vi "GageAdvMultiRec8bit_Core.vi"(5 "Encoder feedback ref":refnum<vi>, 8 "error in":errorcluster, 9 "SignalBuffer queue in":refnum<queue>, 10 "GenericDAQ CtrlQueue in":refnum<queue>) -> (0 "error out":errorcluster)   [LabVIEW 2014]
uses:
  <instrlib>/GenericDAQ/VI/GenericDAQ_Ctrl_Queue.ctl
  <instrlib>/GenericDAQ/VI/GenericDAQ_State.ctl
  <instrlib>/GenericDAQ/VI/GenericDAQ_Signal.ctl
  <instrlib>/GageLv_uic/VI/Gage_Configs.ctl
  <instrlib>/GageLv_uic/VI/Gage_PrivateStats.ctl
  <instrlib>/GageLv_uic/VI/Gage_DAQStatus.ctl
  EncoderReadout/VI/EncoderReadout_PrivateStats.ctl
  EncoderReadout/VI/Encoder_State.ctl
  <instrlib>/GageLv_uic/VI/SetSecondaryDataVIRef_Typedef.ctl
  <vilib>/Utility/error.llb/Error Cluster From Error Code.vi
  <vilib>/ErrorRing/Error Ring.xnode
  <instrlib>/GageLv_uic/GageLv.lvlib
  <userlib>/Utility/ErrorLog_lib.lvlib
  EncoderReadout/EncoderReadout(NI-DAQmx).lvlib
  <instrlib>/GenericDAQ/GenericDAQ.lvlib
panel:
  out "element":T1
  out "Segment Count (1)":u32
  out "GenericDAQ State":T2
  out "ctrl elements":T3[](array[typedef])
  out "DynamicBuffer_Bak":refnum<queue>
  in  "SetPosition":dbl[](array[numeric])=[0.0, 0.0]
  out "pos_raw_data":dbl[][](array[numeric])
  out "volt conv. time":u32
  out "transfer time":u32
  in  "StartAll":bool
  in  "Get_ConfigAll":bool
  out "LiveStat":T4
  in  "Gage_Config":T6={"Acquisition"={"Sample Rate"=4000000000.0, "Mode"=0, "Start (0)"=0.0, "Depth"=8192.0, "Segment Size"=8192.0, "Trigger Delay"=0.0, "Trigger Timeout"=10.0, "Trigger Holdoff"=0.0, "Clock mode"=enum."Internal", "Segment"=1}, "Channels"=[{"Coupling"=0, "Differential Input"=FALSE, "Direct-to-ADC"=FALSE, "Range"=2000, "Impedance"=50, "DC Offset"=0, "Filter"=0}], "Trigger"={"Slope"=0, "Level"=25, "Source"=0, "External Range"=2000, "External Coupling"=0, "External"=TRUE, "Disable"=FALSE, "External Impedance"=0}, "Mode(Gage)"=enum."Continuous"} {"Trigger"."External Impedance" items=["50 Ohm", "HiZ"]; "Trigger"."External Coupling" items=["DC", "AC"]; "Trigger"."External Range" min=2000 max=10000 step=8000; "Trigger"."Slope" items=["Rising", "Falling"]; "Trigger"."Level" min=-100 max=100; "Trigger"."Source" min=0 max=64 step=1; "Channels"."Impedance" min=50 max=1000000 step=999950; "Channels"."Coupling" items=["DC", "AC"]; "Acquisition"."Start (0)" min=-1000000.0 max=0.0 step=16.0; "Acquisition"."Segment Size" min=256.0 step=128.0; "Acquisition"."Trigger Delay" min=0.0 step=128.0; "Acquisition"."Trigger Timeout" format="%.0p"; "Acquisition"."Trigger Holdoff" min=0.0 step=128.0; "Acquisition"."Depth" min=256.0 step=128.0; "Acquisition"."Mode" items=["Single", "Dual", "Quad", "Octal"]; "Acquisition"."Sample Rate" format="%.0p"}
  out "Graph":sgl[](graph)
  in  "fConfig":bool
  in  "Reset":bool
  in  "CloseAll":bool
  in  "Close":bool
  in  "Enumerate":bool
  in  "Open":bool
  in  "Quit":bool
  in  "Start":bool
  in  "ConfigAll":bool
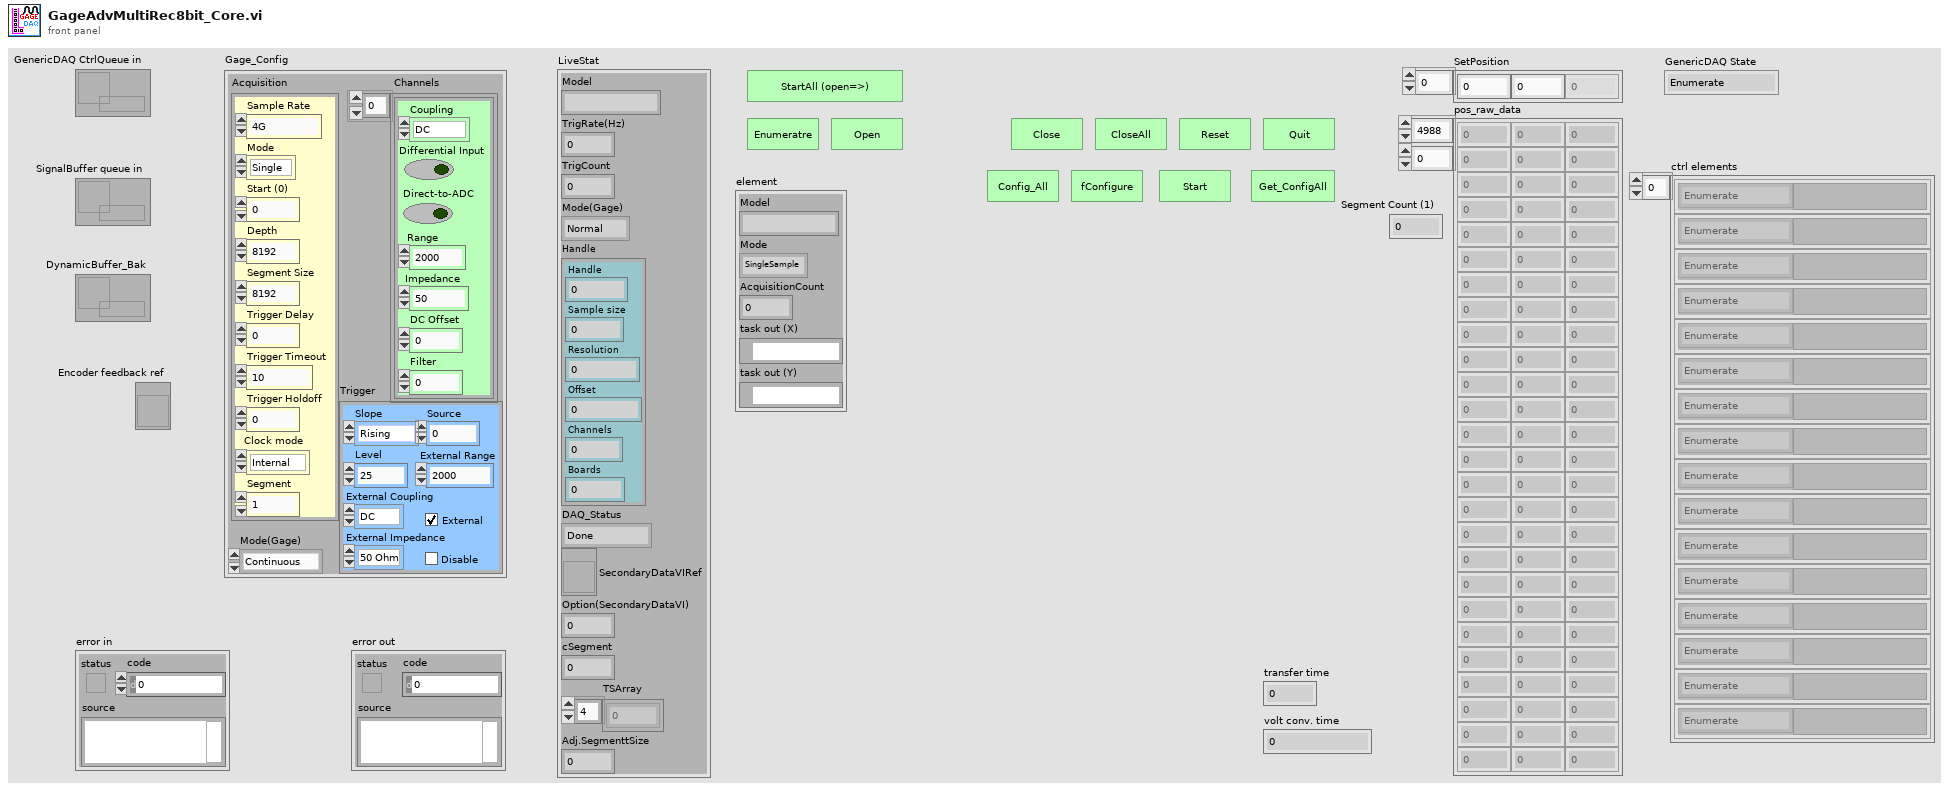
[diagram p1: front panel]
types:
  T1 = typedef "EncoderReadout(NI-DAQmx).lvlib/EncoderReadout_PrivateStats.ctl" = cluster{"Model":string, "Mode":enum16{"SingleSample", "NSamples", "Continuous"}, "AcquisitionCount":i32, "task out (X)":refnum<k21>, "task out (Y)":refnum<k21>}
  T2 = typedef "GenericDAQ.lvlib/GenericDAQ_State.ctl" = enum16{"Enumerate", "Open", "Close", "CloseAll", "Reset", "Quit", "==Settings==", "SetAcquisition_", "SetChannels_", "SetTrigger_", "SetAnalogTrigDetector_", "SetSegment#_", "SetAll_AcquChTrig_", "fConfigurate", "fStart", "GetStatus", "_WaitForDone/Idle", "_GetData", "GetAcquisition", "GetChannels", "GetTrigger", "GetAll_AcquChTrig", "Abort", "==Messaging==", "_PushDataOut", "GetStat_", "GetConfig_", "==ModeSetup==", "SetSignalBuffer_", "SetMode_", "SetSecondaryDataRef._", "SetDynamicBuffer_", "==AnalogOut==", "GetChannelCount_AO", "fStart_AO", "SetChEnable_AO", "SetConfig_AO", "SetFuncData_AO", "SetOffset_AO_", "SetMasterNode_AO", "SetStates_AO", "SetSymetry_AO", "SetTriggerSource_AO", "==Trigger==", "ManualTrigger", "===Sync===", "LineStart", "LineEnd", "FrameStart", "FrameEnd", "EOL_PassThrough", "SOL_PassThrough"}
  T3 = typedef "GenericDAQ.lvlib/GenericDAQ_Ctrl_Queue.ctl" = cluster{"GenericDAQ State":T2, "Variant":variant}
  T4 = typedef "GageLv.lvlib/Gage_PrivateStats.ctl" = cluster{"Model":string, "TrigRate(Hz)":dbl, "TrigCount":i32, "Mode(Gage)":enum16{"Normal", "Continuous", "MultiRecord", "HwAverage"}, "Handle":cluster{"Handle":u32, "Sample size":u32, "Resolution":i32, "Offset":i32, "Channels":u32, "Boards":u32}, "DAQ_Status":T5, "SecondaryDataVIRef":refnum<vi>, "Option(SecondaryDataVI)":i32, "cSegment":i32, "TSArray":dbl[], "Adj.SegmenttSize":dbl}
  T5 = typedef "GageLv.lvlib/Gage_DAQStatus.ctl" = enum16{"Done", "Armed", "Triggered", "Transfering"}
  T6 = typedef "GageLv.lvlib/Gage_Configs.ctl" = cluster{"Acquisition":cluster{"Sample Rate":dbl, "Mode":u16, "Start (0)":dbl, "Depth":dbl, "Segment Size":dbl, "Trigger Delay":dbl, "Trigger Timeout":dbl, "Trigger Holdoff":dbl, "Clock mode":enum16{"Internal", "External", "Reference"}, "Segment":u32}, "Channels":cluster{"Coupling":u16, "Differential Input":bool, "Direct-to-ADC":bool, "Range":u32, "Impedance":u32, "DC Offset":i32, "Filter":i32}[], "Trigger":cluster{"Slope":u16, "Level":i32, "Source":i32, "External Range":u32, "External Coupling":u16, "External":bool, "Disable":bool, "External Impedance":u16}, "Mode(Gage)":enum16{"Normal", "Continuous", "MultiRecord", "HwAverage"}}
  T7 = typedef "SetSecondaryDataVIRef_Typedef.ctl" = cluster{"SecondaryDataVIRef.":refnum<vi>, "Option":i32}
  T8 = cluster{"tickcount":u32, "Position":dbl[][], "Flag":enum16{"Normal", "MultiRecStart", "MultiRecEnd", "Reserved1", "Reserved2", "Reserved3"}}
  T9 = typedef "EncoderReadout(NI-DAQmx).lvlib/Encoder_State.ctl" = cluster{"EncoderReadout States":enum16{"Open", "Close", "Quit", "SetPosition", "SetPointsNum", "SetSyncChannel", "Start(Flush)", "GetPositions", "QueryStatus", "SetTimeout", "SetMode", "SetSignalOutputBuffer", "GetConfigs", "Wait", "Clear", "Stop", "FlushBuffer"}, "Variant":variant}
  T10 = typedef "GenericDAQ.lvlib/GenericDAQ_Signal.ctl" = cluster{"tickcount":u32, "Signal":sgl[], "SecondaryData":dbl[], "Flag":enum16{"Normal", "LineStart", "LineEnd", "FrameStart", "FrameEnd", "Reserved1", "Reserved2"}, "Segment#":i32}
  T11 = enum16{"Normal", "LineStart", "LineEnd", "FrameStart", "FrameEnd", "Reserved1", "Reserved2"}
  T12 = enum16{"Normal", "Continuous", "MultiRecord", "HwAverage"}
  T13 = cluster{"Handle":u32, "Sample size":u32, "Resolution":i32, "Offset":i32, "Channels":u32, "Boards":u32}
  T14 = cluster{"Sample Rate":dbl, "Mode":u16, "Start (0)":dbl, "Depth":dbl, "Segment Size":dbl, "Trigger Delay":dbl, "Trigger Timeout":dbl, "Trigger Holdoff":dbl, "Clock mode":enum16{"Internal", "External", "Reference"}, "Segment":u32}
  T15 = cluster{"Sample Rate":dbl, "Clock mode":enum16{"Internal", "External", "Reference"}, string, "Depth":dbl, "Segment Size":dbl, "Trigger Timeout":dbl, "Trigger Holdoff":dbl, "Trigger Delay":dbl}
  T16 = cluster{"Coupling":u16, "Differential Input":bool, "Direct-to-ADC":bool, "Range":u32, "Impedance":u32, "DC Offset":i32, "Filter":i32}[]
  T17 = cluster{string, "Differential Input":bool, "Direct-to-ADC":bool, "Range":u32, "Impedance":u32, "DC Offset":i32, "Filter":i32}
  T18 = cluster{"Slope":u16, "Level":i32, "Source":i32, "External Range":u32, "External Coupling":u16, "External":bool, "Disable":bool, "External Impedance":u16}
  T19 = cluster{string, "Level":i32, "Source":i32, "External Range":u32, string, "External":bool, "Disable":bool, string}
  T20 = cluster{string, "Level":i32, "Source":i32, "External Range":u32, string, "External":bool, "Disable":bool, string}[]
  T21 = cluster{"Handle":u32, "Sample Size":u32, "Resolution":i32, "Offset":i32, "Channels":u32, "Boards":u32}
  T22 = cluster{"Coupling":u16, "Differential Input":bool, "Direct-to-ADC":bool, "Range":u32, "Impedance":u32, "DC Offset":i32, "Filter":i32}
  T23 = cluster{"queue out":refnum<queue>, "queue out":refnum<queue>}
  T24 = typedef "Gage.lvlib/Gage_Configs.ctl" = cluster{"Acquisition":cluster{"Sample Rate":dbl, "Mode":u16, "Start (0)":dbl, "Depth":dbl, "Segment Size":dbl, "Trigger Delay":dbl, "Trigger Timeout":dbl, "Trigger Holdoff":dbl, "Clock mode":enum16{"Internal", "External", "Reference"}, "Segment":u32}, "Channels":cluster{"Coupling":u16, "Differential Input":bool, "Direct-to-ADC":bool, "Range":u32, "Impedance":u32, "DC Offset":i32, "Filter":i32}[], "Trigger":cluster{"Slope":u16, "Level":i32, "Source":i32, "External Range":u32, "External Coupling":u16, "External":bool, "Disable":bool, "External Impedance":u16}, "Mode(Gage)":enum16{"Normal", "Continuous", "MultiRecord", "HwAverage"}}
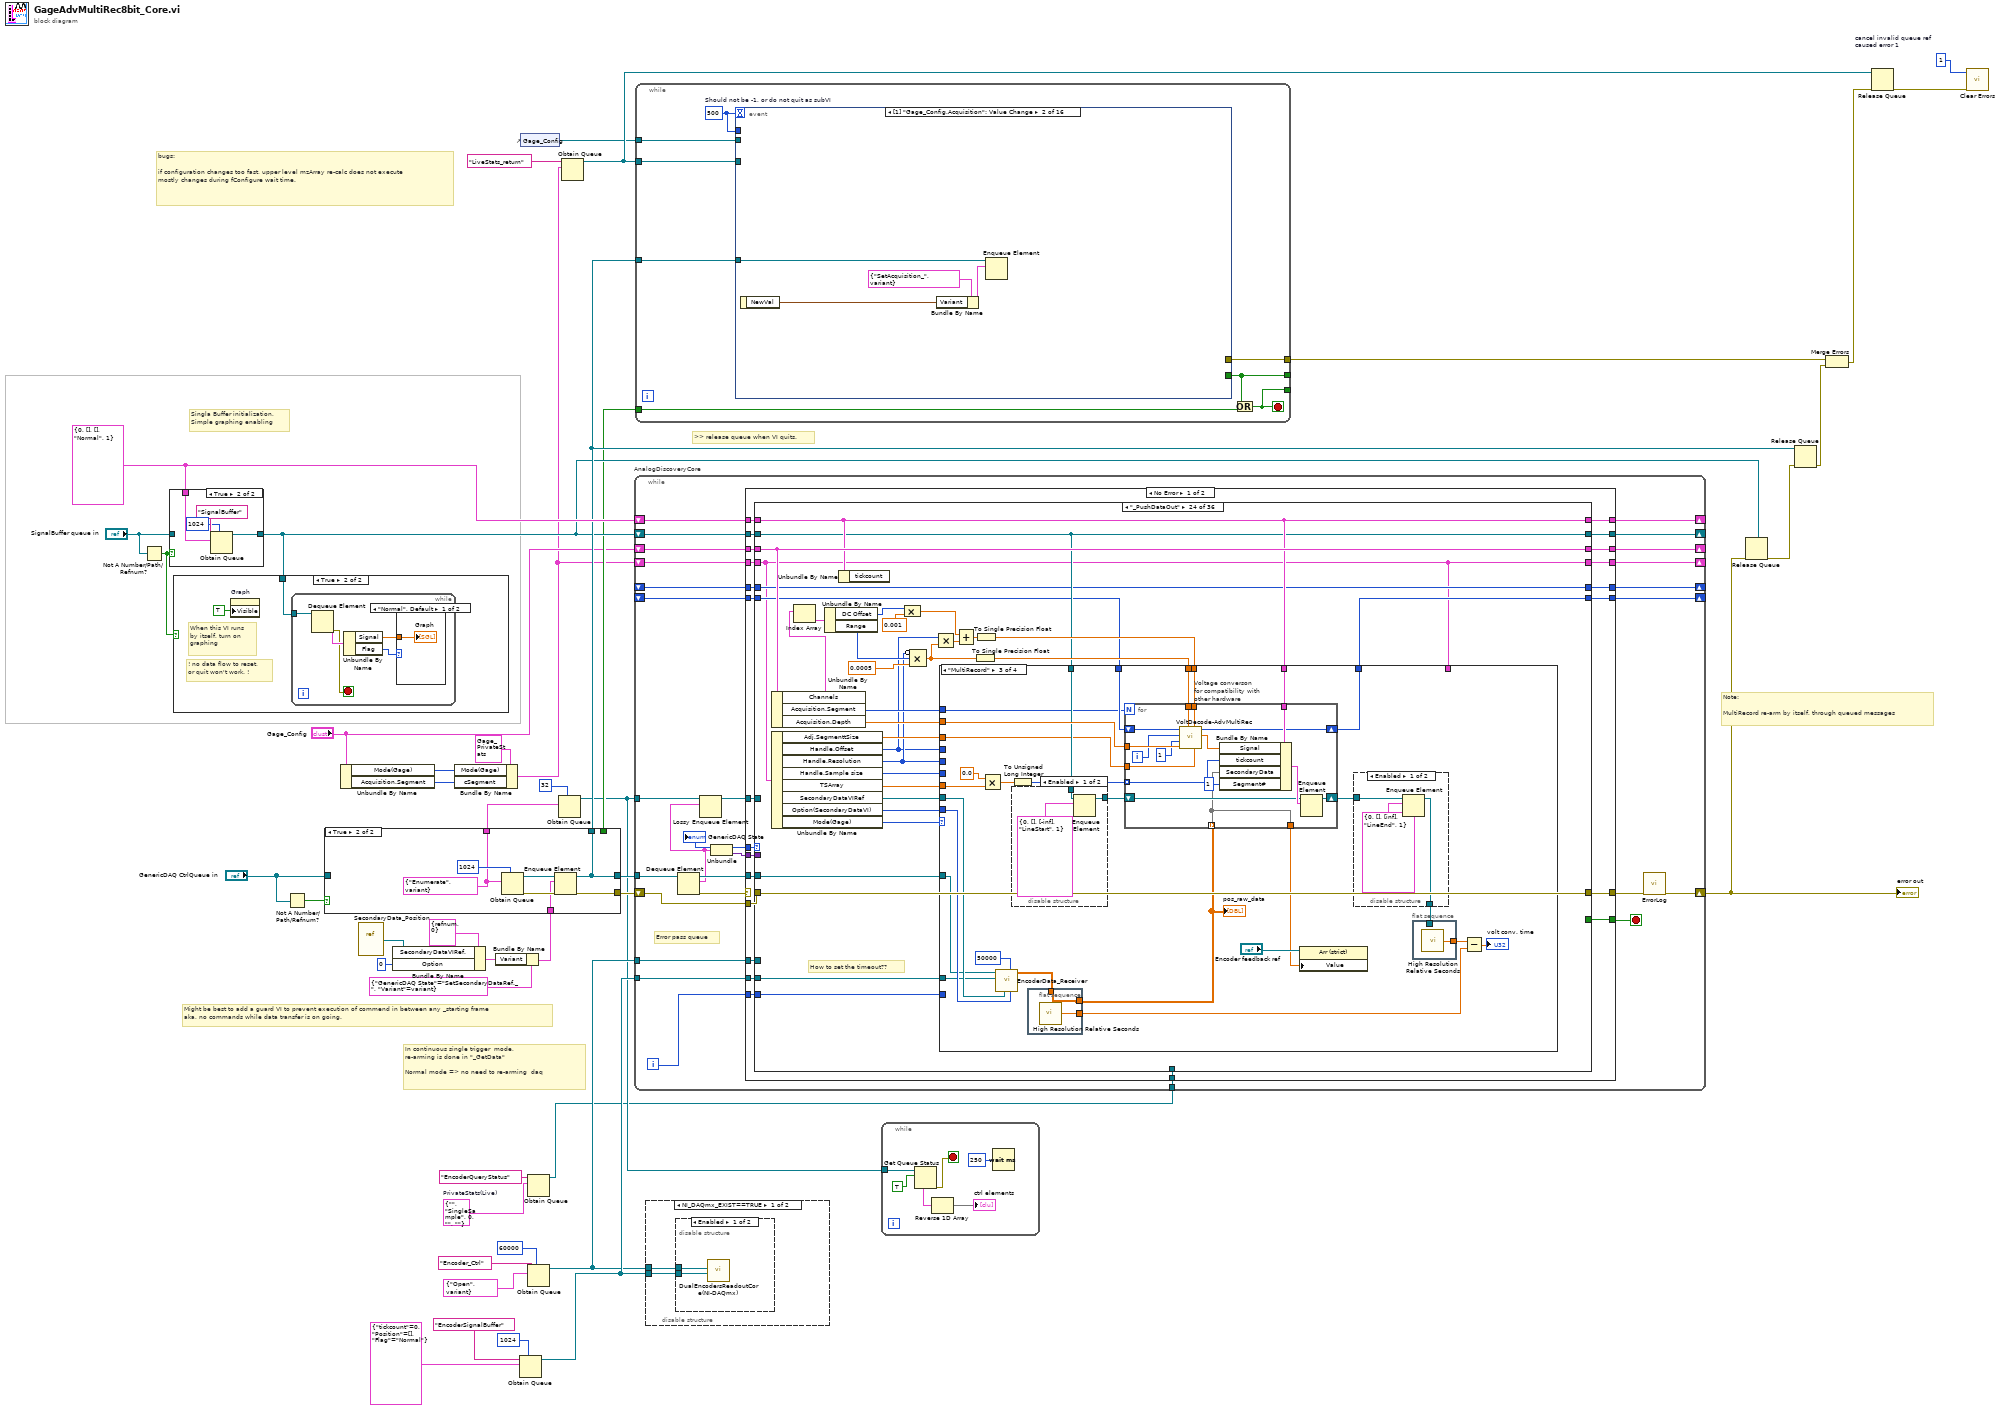
[diagram p0: block diagram]
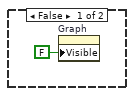
[diagram p4: hidden frame]
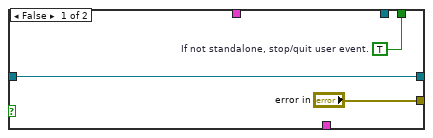
[diagram p7: hidden frame]
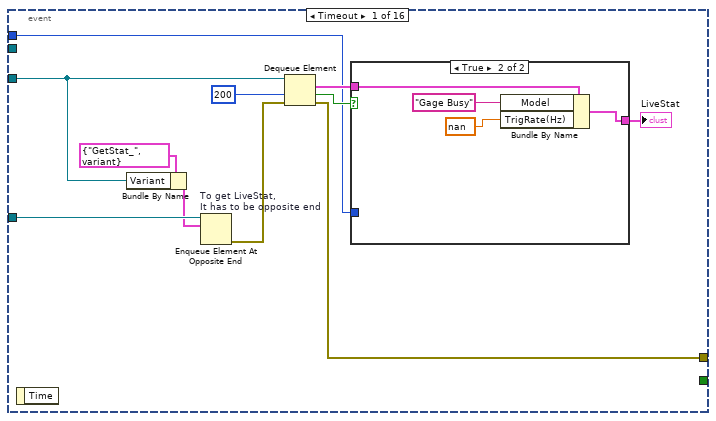
[diagram p8: hidden frame]
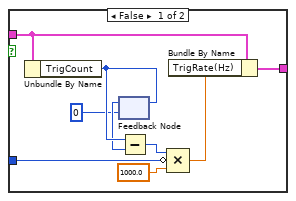
[diagram p9: hidden frame]
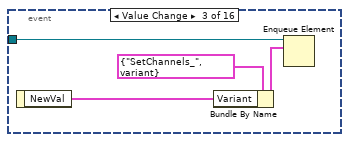
[diagram p10: hidden frame]
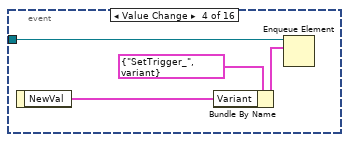
[diagram p11: hidden frame]
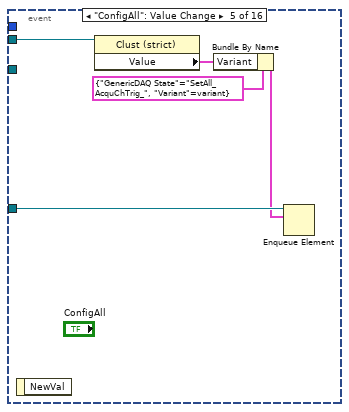
[diagram p12: hidden frame]
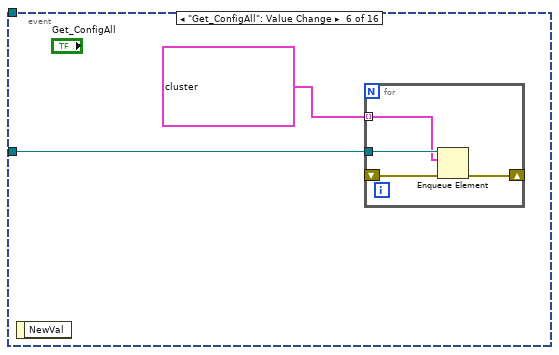
[diagram p13: hidden frame]
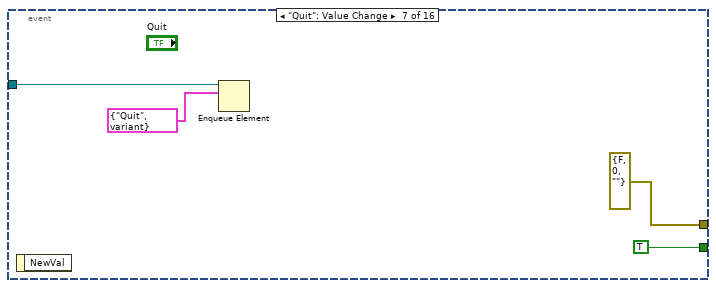
[diagram p14: hidden frame]
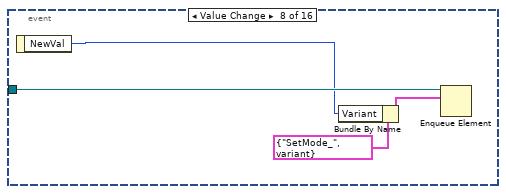
[diagram p15: hidden frame]
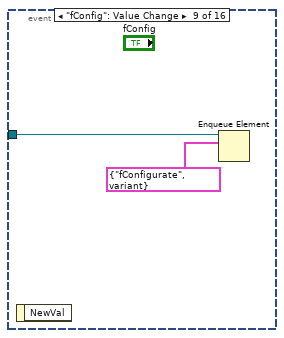
[diagram p16: hidden frame]
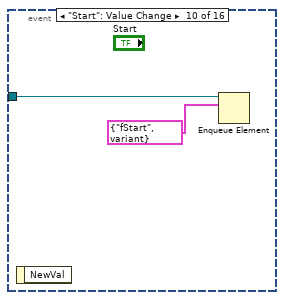
[diagram p17: hidden frame]
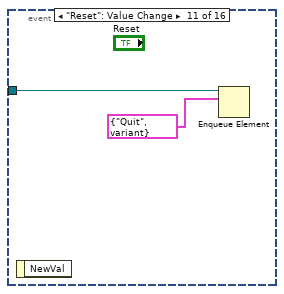
[diagram p18: hidden frame]
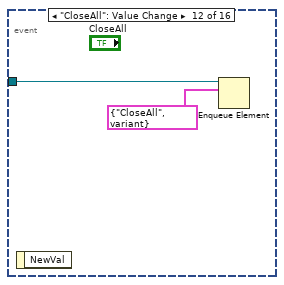
[diagram p19: hidden frame]
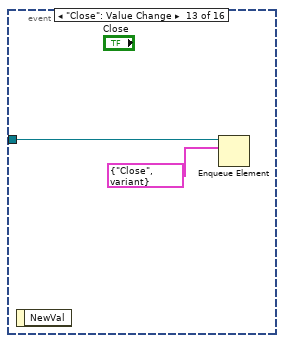
[diagram p20: hidden frame]
diagram:
  w3 = T1 {"Model"="", "Mode"=enum."SingleSample", "AcquisitionCount"=0, "task out (X)"="", "task out (Y)"=""}  # PrivateStats(Live)
  w29 = 1  # cancel invalid queue ref caused error 1
  w45 = T10 {"tickcount"=0, "Signal"=[], "SecondaryData"=[], "Flag"=enum."Normal", "Segment#"=1} ("Signal_Typedef")
  # "Note:\n\nMultiRecord re-arm by itself, through queued messages"
  # "In continuous single trigger  mode, \nre-arming is done in \"_GetData\"\n\nNormal mode => no need to re-arming  daq"
  # "Might be best to add a guard VI to prevent execution of commend in between any _starting frame \naka, no commands while data transfer is on going."
  # "bugs:\n\nif configuration changes too fast, upper level mzArray re-calc does not execute\nmostly changes during fConfigure wait time."
  # "Singla Buffer initialization,\nSimple graphing enabling"
  # ">> release queue when VI quits."
  n1 = Not A Number/Path/Refnum?(number/path/refnum="SignalBuffer queue in") -> (NaN/Path/Refnum?=w32:bool)
  n2 = case shown="True" w32 {
    tunnel: w45 -> [_ w50]
    tunnel: [w46 w49] -> w33
    tunnel: "SignalBuffer queue in" -> [w46 _]
    frame False {
    }
    frame True {
      n3 = Obtain Queue(max queue size (-1, unlimited)=1024, name (unnamed)="SignalBuffer", element data type=w50) -> (queue out=w49:refnum<queue>)  [unwired: 2 in, 2 out]
    }
  }
  n4 = case shown="True" w32 {
    tunnel: w33 -> [_ w53]
    frame False {
      n5 = property on="Graph" class="WFGraph (strict)"("Visible"=FALSE) -> ()  [unwired: 2 in, 2 out]
    }
    frame True {
      # "! no data flow to reset,\nor quit won't work. !"
      # "When this VI runs\nby itself, turn on \ngraphing"
      n6 = property on="Graph" class="WFGraph (strict)"("Visible"=TRUE) -> ()  [unwired: 2 in, 2 out]
      n7 = while {
        tunnel: w53 -> [w58]
        stop <- w55 stop-if-true
        n8 = Dequeue Element(queue=w58) -> (element=w57:T10, error out=w55:errorcluster)  [unwired: 2 in, 2 out]
        n9 = Unbundle By Name(w57) -> ("Signal"=w56:sgl[], "Flag"=w54:T11)
        n10 = case shown="\"Normal\", Default" w54 {
          tunnel: w56 -> [w59 _]
          frame "Normal", Default {
            "Graph" <- w59
          }
          frame "LineStart", "LineEnd" {
          }
        }
      }
    }
  }
  n11 = Not A Number/Path/Refnum?(number/path/refnum="GenericDAQ CtrlQueue in") -> (NaN/Path/Refnum?=w42:bool)
  n12 = Unbundle By Name("Gage_Config") -> ("Mode(Gage)"=w25:T12, "Acquisition.Segment"=w19:u32)
  n13 = vi-ref "SecondaryData_Position.vi"() -> (w8:refnum<vi>)
  n14 = Bundle By Name(cluster=T7 {"SecondaryDataVIRef."=refnum, "Option"=0} ("SecondaryDataParams."), "SecondaryDataVIRef."=w8, "Option"=0) -> (w6:T7)
  n15 = Bundle By Name(cluster=T4 {"Model"="", "TrigRate(Hz)"=0.0, "TrigCount"=0, "Mode(Gage)"=enum."Normal", "Handle"={"Handle"=0, "Sample size"=0, "Resolution"=0, "Offset"=0, "Channels"=0, "Boards"=0}, "DAQ_Status"=enum."Done", "SecondaryDataVIRef"=refnum, "Option(SecondaryDataVI)"=0, "cSegment"=0, "TSArray"=[], "Adj.SegmenttSize"=0.0} ("PrivateStats(Live)"), "Mode(Gage)"=w25, "cSegment"=w19) -> (w22:T4)
  n16 = Bundle By Name(cluster=T3 {"GenericDAQ State"=enum."SetSecondaryDataRef._", "Variant"=variant} ("element"), "Variant"=w6) -> (w5:T3)
  n17 = case shown="True" w42 {
    tunnel: [w62 w66] -> w44
    tunnel: ["error in" w65] -> w43
    tunnel: "GenericDAQ CtrlQueue in" -> [w62 _]
    tunnel: [_ w66] -> w38
    tunnel: [w60 _] -> w28
    tunnel: [_ w68] -> w21
    tunnel: w5 -> [_ w63]
    frame False {
      w60 = TRUE  # If not standalone, stop/quit user event.
    }
    frame True {
      w68 = T3 {"GenericDAQ State"=enum."Enumerate", "Variant"=variant}
      n18 = Obtain Queue(max queue size (-1, unlimited)=1024, element data type=w68) -> (queue out=w67:refnum<queue>, error out=w64:errorcluster)  [unwired: 3 in, 1 out]
      n19 = Enqueue Element(queue=w67, element=w63, error in (no error)=w64) -> (queue out=w66:refnum<queue>, error out=w65:errorcluster)  [unwired: 1 in, 1 out]
    }
  }
  n20 = Obtain Queue(max queue size (-1, unlimited)=1024, name (unnamed)="EncoderSignalBuffer", element data type=T8 {"tickcount"=0, "Position"=[], "Flag"=enum."Normal"} ("Signal_Typedef")) -> (queue out=w12:refnum<queue>)  [unwired: 2 in, 2 out]
  n21 = control-ref of="Gage_Config"() -> (w23:refnum<vi>)
  n22 = Obtain Queue(name (unnamed)="EncoderQueryStatus", element data type=w3) -> (queue out=w1:refnum<queue>)  [unwired: 3 in, 2 out]
  n23 = Obtain Queue(max queue size (-1, unlimited)=60000, name (unnamed)="Encoder_Ctrl", element data type=T9 {"EncoderReadout States"=enum."Open", "Variant"=variant}) -> (queue out=w11:refnum<queue>)  [unwired: 2 in, 2 out]
  n24 = Obtain Queue(max queue size (-1, unlimited)=32, element data type=w21) -> (queue out=w4:refnum<queue>)  [unwired: 3 in, 2 out]
  n25 = Obtain Queue(name (unnamed)="LiveStats_return", element data type=w22) -> (queue out=w36:refnum<queue>)  [unwired: 3 in, 2 out]
  n26 = while "AnalogDiscoveryCore" {
    shift-right: [w96] -> _
    shift-left: w33 -> [w97]
    tunnel: w44 -> [w85]
    shift-right: [w71] -> w31
    shift-left: w43 -> [w87]
    shift-right: [w94] -> _
    shift-left: "Gage_Config" -> [w93]
    shift-right: [w79] -> _
    shift-left: w22 -> [w92]
    shift-right: [w88] -> _
    shift-left: w45 -> [w91]
    shift-right: [w82] -> _
    shift-left: _ -> [w80]
    shift-right: [w83] -> _
    shift-left: _ -> [w81]
    tunnel: w4 -> [w74]
    tunnel: w11 -> [w77]
    tunnel: w12 -> [w76]
    tunnel: w1 -> [w70]
    i -> [w75]
    stop <- w95 stop-if-true
    # "Error pass queue"
    n27 = Dequeue Element(queue=w85) -> (queue out=w84:refnum<queue>, element=w73:T3, error out=w86:errorcluster)  [unwired: 2 in, 1 out]
    n28 = Lossy Enqueue Element(queue=w74, element=w73) -> (queue out=w72:refnum<queue>)  [unwired: 1 in, 3 out]
    n29 = Unbundle(w73) -> ("GenericDAQ State"=w90:T2, "Variant"=w89:variant)
    "GenericDAQ State" <- w90
    n30 = case shown="No Error" w86 {
      tunnel: w97 -> [w120 w1276]
      tunnel: [w119 w1276] -> w96
      tunnel: [w118 TRUE] -> w95
      tunnel: [w117 w1274] -> w78
      tunnel: [w116 w1277] -> w94
      tunnel: w93 -> [w115 w1277]
      tunnel: w92 -> [w114 w1278]
      tunnel: w91 -> [w113 w1275]
      tunnel: w84 -> [w112 _]
      tunnel: w90 -> [w111 _]
      tunnel: w89 -> [w110 _]
      tunnel: [w109 w1275] -> w88
      tunnel: [w108 w1278] -> w79
      tunnel: w87 -> [w107 _]
      tunnel: [w106 w1273] -> w83
      tunnel: [w105 w1272] -> w82
      tunnel: w81 -> [w104 w1273]
      tunnel: w80 -> [w103 w1272]
      tunnel: w77 -> [w102 _]
      tunnel: w76 -> [w101 _]
      tunnel: w75 -> [w100 _]
      tunnel: w72 -> [w99 _]
      tunnel: w70 -> [w98 _]
      frame No Error {
        n31 = case shown="\"_PushDataOut\"" w111 {
          tunnel: w120 -> [w128 w172 w189 w204 w223 w242 w259 w280 w340 w394 w454 w514 w558 w591 w648 w674 w729 w814 w828 w870 w880 w903 w936 w956 w1074 w1086 w1098 w1111 w1138 w1163 w1191 w1217 w1218 w1227 w1244 w1271]
          tunnel: [w128 w172 w189 w204 w223 w242 w259 w280 w340 w394 w454 w514 w558 w591 w648 w674 w729 w814 w828 w870 w880 w903 w936 w956 w1074 w1086 w1098 w1112 w1138 w1163 w1192 w1217 w1218 w1227 w1244 w1271] -> w119
          tunnel: [_ _ _ _ _ w237 _ _ _ _ _ _ _ _ _ _ _ _ _ _ _ _ _ _ _ _ _ _ _ _ _ _ _ _ _ _] -> w118
          tunnel: w112 -> [_ _ _ _ w220 w234 _ w269 w329 w383 w443 w512 w543 w573 _ w676 w726 _ _ _ w874 w898 _ w973 _ _ _ _ _ _ _ _ _ _ _ _]
          tunnel: w107 -> [w124 w168 w184 w203 w219 w235 _ w274 w333 w387 w448 w506 w548 w575 w645 w675 w724 w813 w827 w869 w873 w897 _ w974 w1069 w1078 _ w1108 w1129 _ _ w1216 w1225 w1233 w1243 w1270]
          tunnel: [w124 w150 w179 w197 w218 w236 w255 w265 w334 w388 w442 w511 w546 w583 w645 w669 w713 w792 w817 w845 w872 w896 w932 w974 w1068 w1079 w1094 w1109 w1130 w1152 w1194 w1216 w1225 w1233 w1243 w1270] -> w117
          tunnel: [w127 w171 w188 w202 w222 w241 w258 w277 w327 w381 w451 w509 w557 w590 w647 w673 w730 w809 w824 w863 w877 w902 w935 w972 w1067 w1080 w1097 w1116 w1137 w1162 w1201 w1215 w1224 w1232 w1242 w1269] -> w116
          tunnel: w115 -> [w127 w171 w188 w202 w222 w241 w258 w275 w328 w382 w449 w509 w557 w590 w647 w673 w730 w811 w822 w868 w877 w902 w935 w972 w1067 w1080 w1097 w1116 w1137 w1162 w1201 w1215 w1224 w1232 w1242 w1269]
          tunnel: [w126 w164 w185 w198 w217 w239 w257 w278 w338 w392 w452 w503 w555 w579 w644 w667 w711 w805 w823 w864 w879 w892 w934 w942 w1064 w1085 w1096 w1115 w1135 w1158 w1193 w1214 w1223 w1231 w1238 w1268] -> w108
          tunnel: w114 -> [w126 w169 w186 w198 w217 w239 w257 w278 w338 w392 w452 w503 w555 w579 w640 w668 w722 w810 w823 w864 w879 w892 w934 w942 w1064 w1085 w1096 w1115 w1134 w1153 w1193 w1214 w1223 w1231 w1238 w1268]
          tunnel: w113 -> [w125 w170 w187 w201 w221 w240 w256 w279 w339 w393 w453 w513 w556 w589 w646 w672 w728 w812 w826 w867 w878 w901 w933 w971 w1073 w1084 w1095 w1114 w1136 w1161 w1200 w1213 w1222 w1230 w1241 w1267]
          tunnel: w110 -> [_ w167 _ _ _ _ _ w276 w337 w391 w450 w510 _ _ _ _ _ _ _ _ _ _ _ _ w1070 w1083 _ w1113 w1133 w1156 w1197 _ _ _ _ _]
          tunnel: [w125 w170 w187 w201 w221 w240 w256 w279 w339 w393 w453 w513 w556 w589 w646 w672 w727 w812 w826 w867 w878 w901 w933 w971 w1073 w1084 w1095 w1114 w1136 w1161 w1200 w1213 w1222 w1230 w1241 w1267] -> w109
          tunnel: [w122 w155 w183 w200 w211 w233 w254 w272 w331 w385 w446 w505 w553 w586 w643 w657 w703 w799 w819 w866 w876 w900 w931 w950 w1066 w1077 w1093 w1105 w1128 w1160 w1199 w1212 w1221 w1229 w1240 w1266] -> w106
          tunnel: [w121 w154 w182 w199 w210 w232 w253 w271 w330 w384 w445 w504 w552 w585 w642 w656 w702 w798 w818 w865 w875 w899 w930 w951 w1065 w1076 w1092 w1104 w1127 w1159 w1198 w1211 w1220 w1228 w1239 w1265] -> w105
          tunnel: w104 -> [w122 _ w183 w200 w211 w233 w254 w272 w331 w385 w446 w505 w553 w586 w643 w657 w705 w799 w819 w866 w876 w900 w931 w950 w1066 w1077 w1093 w1105 w1128 w1160 w1199 w1212 w1221 w1229 w1240 w1266]
          tunnel: w103 -> [w121 _ w182 w199 w210 w232 w253 w271 w330 w384 w445 w504 w552 w585 w642 w656 w704 w798 w818 w865 w875 w899 w930 w953 w1065 w1076 w1092 w1104 w1127 w1159 w1198 w1211 w1220 w1228 w1239 w1265]
          tunnel: w102 -> [_ w140 w176 _ w205 w229 _ w270 _ _ w444 _ _ w581 _ _ _ _ _ _ _ w885 _ _ _ _ _ _ w1122 _ _ _ _ _ w1234 _]
          tunnel: w101 -> [_ _ _ _ _ _ _ _ _ _ _ _ _ w576 _ _ _ _ _ _ _ _ _ w954 _ _ _ _ _ _ _ _ _ _ _ _]
          tunnel: w100 -> [_ _ _ _ _ _ _ _ _ _ _ _ _ _ _ _ _ _ _ _ _ _ _ w947 _ _ _ _ _ _ _ _ _ _ _ _]
          tunnel: w99 -> [_ _ _ _ _ w228 _ _ _ _ _ _ _ _ _ _ _ _ _ _ _ _ _ _ _ _ _ _ _ _ _ _ _ _ _ _]
          tunnel: w98 -> [_ _ _ _ _ _ _ _ _ _ _ _ _ w569 _ _ _ _ _ _ _ _ _ _ _ _ _ _ _ _ _ _ _ _ _ _]
          frame "Enumerate" {
            n32 = call <instrlib>:"CsTool-Initialize.vi"() -> ("Number Of Systems"=w123:i32)  [unwired: 1 out]
            n33 = call <instrlib>:"CsTool-ErrorHandler.vi"("Error Code"=w123) -> ()  [unwired: 2 in, 1 out]
          }
          frame "Open" {
            w153 = 268435456  # 2GB default
            w156 = u8 0  # 8-bit
            w157 = i16 0  # 16-bit
            w149 = 1  # 1ch default
            # "resevered for future"
            # "Set to valid onboard RAM size:\n256MB : 268435456\n512B : 536870912\n1GB : 1073741824 \n2GB : 2147483648 \n4GB : 4294967296"
            n34 = Variant To Data(error in=w168, type="", Variant=w167) -> (data=w163:string, error out=w131:errorcluster)
            n35 = Select(t="any", s=TRUE, f=w163) -> (s? t:f=w162:string)
            n36 = property on="Segment" class="DigNum (strict)"() -> ("Value"=w134:u32)  [unwired: 2 in, 2 out]
            n37 = call <instrlib>:"CsTool-GetSystem.vi"("Board Name (Any)"=w162) -> ("Error Code"=w165:i32, "Handle Cluster"=w151:T13)  [unwired: 3 in]
            n38 = Bundle By Name(cluster=T9 {"EncoderReadout States"=enum."SetSyncChannel", "Variant"=variant}, "Variant"=tag "/cDAQ1Mod3/PFI3" ("SyncSource")) -> (w145:T9)
            n39 = Bundle By Name(cluster=T9 {"EncoderReadout States"=enum."SetTimeout", "Variant"=variant}, "Variant"=300.0 ("Timeout (s)")) -> (w146:T9)
            n40 = Bundle By Name(cluster=T9 {"EncoderReadout States"=enum."SetPointsNum", "Variant"=variant}, "Variant"=w134) -> (w133:T9)
            n41 = Bundle By Name(cluster=T9 {"EncoderReadout States"=enum."SetPosition", "Variant"=variant}, "Variant"="SetPosition") -> (w132:T9)
            n42 = call <instrlib>:"CsTool-GetSystemName.vi"("Handle Cluster"=w151) -> ()  [unwired: 2 out]
            n43 = call <instrlib>:"CsTool-ErrorHandler.vi"("Error Code"=w165, "Handle Cluster"=w151) -> ("Error String"=w152:string)  [unwired: 1 in]
            n44 = call <instrlib>:"CsTool-GetSystemInfo.vi"("Handle Cluster"=w151) -> ()  [unwired: 7 out]
            n45 = Bundle By Name(cluster=w169, "Handle"=w151, "Model"=w162, "TrigRate(Hz)"=0.0, "TrigCount"=0) -> (w164:T4)
            n46 = Build Array(T9 {"EncoderReadout States"=enum."Open", "Variant"=variant}, w145, w146, w133, w132) -> (w141:T9[])
            n47 = for {
              shift-right: [w174] -> _
              shift-left: w140 -> [w175]
              tunnel: w141 -> [w173] mode=indexing
              n48 = Enqueue Element(queue=w175, element=w173) -> (queue out=w174:refnum<queue>)  [unwired: 2 in, 2 out]
            }
            n49 = Quotient & Remainder(x=w153, y=w149) -> (floor(x/y)=w147:i32)  [unwired: 1 out]
            n50 = call <vilib>:"Clear Errors.vi"("error in (no error)"=w131, "specific error code to clear (0: all)"=91) -> ("error out"=w130:errorcluster)  [unwired: 4 in, 1 out]
            n51 = Bundle By Name(cluster=w130, "source"=w152) -> (w150:errorcluster)
            n52 = Initialize Array(w157, 0 ("dimension size")) -> (w155:i16[])
            n53 = Initialize Array(w156, w147) -> (w154:u8[])
          }
          frame "Close" {
            n54 = Unbundle By Name(w186) -> ("Handle"=w180:T13)
            n55 = Enqueue Element(queue=w176, element=T9 {"EncoderReadout States"=enum."Close", "Variant"=variant}) -> ()  [unwired: 2 in, 3 out]
            n56 = call <instrlib>:"CsTool-AbortCapture.vi"("Handle Cluster"=w180) -> ("Error Code"=w181:i32)
            n57 = call <instrlib>:"CsTool-ErrorHandler.vi"("Error Code"=w181, "Handle Cluster"=w180) -> ("Error String"=w178:string)  [unwired: 1 in]
            n58 = Bundle By Name(cluster=w184, "source"=w178) -> (w179:errorcluster)
            n59 = disable-structure shown="Enabled" {
              disable-tunnel: w186 -> [w192 w193]
              disable-tunnel: [w191 w193] -> w185
              frame Enabled {
                n60 = Bundle By Name(cluster=w192, "Handle.Handle"=u32 0) -> (w191:T4)
              }
              frame Disabled {
              }
            }
          }
          frame "CloseAll" {
            # "not really useful here."
            n61 = Unbundle By Name(w198) -> ("Handle"=w196:T13)
            n62 = call <instrlib>:"CsTool-AbortCapture.vi"("Handle Cluster"=w196) -> ("Error Code"=w195:i32)
            n63 = call <instrlib>:"CsTool-ErrorHandler.vi"("Error Code"=w195, "Handle Cluster"=w196) -> ("Error String"=w194:string)  [unwired: 1 in]
            n64 = Bundle By Name(cluster=w203, "source"=w194) -> (w197:errorcluster)
          }
          frame "Reset" {
            n65 = Unbundle By Name(w217) -> ("Model"=w215:string)
            n66 = Enqueue Element(queue=w205, element=T9 {"EncoderReadout States"=enum."Close", "Variant"=variant}) -> (queue out=w207:refnum<queue>, error out=w206:errorcluster)  [unwired: 2 in, 1 out]
            n67 = Bundle By Name(cluster=T3 {"GenericDAQ State"=enum."Open", "Variant"=variant} ("element"), "Variant"=w215) -> (w214:T3)
            n68 = Build Array(w214, T3 {"GenericDAQ State"=enum."Close", "Variant"=variant} ("element")) -> (w212:T3[])
            n69 = Enqueue Element(queue=w207, element=T9 {"EncoderReadout States"=enum."Open", "Variant"=variant}, error in (no error)=w206) -> ()  [unwired: 1 in, 3 out]
            n70 = for {
              tunnel: w220 -> [w227]
              tunnel: w212 -> [w224] mode=indexing
              shift-right: [w225] -> w218
              shift-left: w219 -> [w226]
              n71 = Enqueue Element At Opposite End(queue=w227, element=w224, error in (no error)=w226) -> (error out=w225:errorcluster)  [unwired: 1 in, 2 out]
            }
          }
          frame "Quit" {
            n72 = Release Queue(queue=w228) -> ()  [unwired: 2 in, 3 out]
            n73 = Unbundle By Name(w239) -> ("Handle"=w231:T13, "Handle.Handle"=w238:u32)
            n74 = case "Check handle leak??" shown="Default" w238 {
              tunnel: [_ TRUE] -> w237
              tunnel: [w244 _] -> w236
              tunnel: w235 -> [w245 _]
              tunnel: w234 -> [w246 _]
              tunnel: w231 -> [_ w251]
              frame Default {
                n75 = for {
                  tunnel: w246 -> [w250]
                  tunnel: T3[] [{"GenericDAQ State"=enum."Quit", "Variant"=variant}, {"GenericDAQ State"=enum."Close", "Variant"=variant}] -> [w247] mode=indexing
                  shift-right: [w248] -> w244
                  shift-left: w245 -> [w249]
                  n76 = Enqueue Element At Opposite End(queue=w250, element=w247, error in (no error)=w249) -> (error out=w248:errorcluster)  [unwired: 1 in, 2 out]
                }
              }
              frame 0 {
                n77 = call <instrlib>:"CsTool-FreeSystem.vi"("Handle Cluster"=w251) -> ()  [unwired: 1 out]
              }
            }
            n78 = Enqueue Element(queue=w229, element=T9 {"EncoderReadout States"=enum."Quit", "Variant"=variant}) -> ()  [unwired: 2 in, 3 out]
          }
          frame "==Settings==" {
            # "Invalid frame"
            n79 = xnode "Error Ring"() -> ("error out"=w255:errorcluster)
          }
          frame "SetAcquisition_" {
            n80 = Unbundle By Name(w275) -> ("Acquisition"=w266:T14)
            n81 = Variant To Data(error in=w274, type=w266, Variant=w276) -> (data=w267:T14, error out=w273:errorcluster)
            n82 = case shown="No Error" w273 {
              selector: w273 -> [w297 _]
              tunnel: w278 -> [w308 _]
              tunnel: w267 -> [w301 _]
              tunnel: [w296 w321] -> w265
              tunnel: w270 -> [w290 _]
              tunnel: w269 -> [w287 _]
              frame No Error {
                n83 = call <instrlib>:"CleanupDAQTasks.vi"("error in (no error)"=w297, "Queue in"=w287) -> ("error out"=w288:errorcluster)  [unwired: 8 in, 1 out]
                n84 = Unbundle By Name(w301) -> ("Segment"=w281:u32, "Mode"=w293:u16, "Sample Rate"=w307:dbl, "Clock mode"=w306:enum16{"Internal", "External", "Reference"})
                n85 = Unbundle By Name(w301) -> ("Depth"=w298:dbl, "Segment Size"=w305:dbl, "Trigger Timeout"=w304:dbl, "Trigger Holdoff"=w303:dbl, "Trigger Delay"=w302:dbl)
                n86 = Unbundle By Name(w308) -> ("Handle"=w295:T13, "Mode(Gage)"=w289:T12)
                n87 = Index Array(array=string[] ["Single", "Dual", "Quad", "Octal"], index=w293) -> (element=w299:string)
                n88 = Scale By Power Of 2(n=w293, x=ext 1.0) -> (x*2^n=w294:ext)
                n89 = To Long Integer(number=w294) -> ()  [unwired: 1 out]
                n90 = Bundle("Sample Rate"=w307, "Clock mode"=w306, w299, "Depth"=w298, "Segment Size"=w305, "Trigger Timeout"=w304, "Trigger Holdoff"=w303, "Trigger Delay"=w302) -> (w286:T15)  [unwired: 1 in]
                n91 = To Long Integer(number=w298) -> ()  [unwired: 1 out]
                n92 = flat-sequence {
                  tunnel: w295 -> [w313]
                  tunnel: [w313] -> w283
                  tunnel: w283 -> [w315]
                  tunnel: [w315] -> w282
                  tunnel: w282 -> [w320]
                  tunnel: w286 -> [w319]
                  tunnel: [w318] -> w285
                  tunnel: [w317] -> w284
                  tunnel: w281 -> [w316]
                  frame #0 {
                    n93 = call <instrlib>:"CsTool-AbortCapture.vi"("Handle Cluster"=w313) -> ()  [unwired: 1 out]
                  }
                  frame #1 {
                    n94 = Wait (ms)(milliseconds to wait=u32 5) -> ()  [unwired: 1 out]
                  }
                  frame #2 {
                    n95 = call <instrlib>:"CsTool-ConfigureAcquisition.vi"("Handle Cluster"=w320, "Segment Count (1)"=w316, "Acquisition"=w319) -> ("Error Code"=w318:i32)  [unwired: 2 in]
                    n96 = call <instrlib>:"CsTool-ErrorHandler.vi"("Error Code"=w318, "Handle Cluster"=w320) -> ("Error String"=w317:string)  [unwired: 1 in]
                  }
                }
                n97 = case shown="\"MultiRecord\"" w289 {
                  tunnel: w290 -> [_ w310]
                  tunnel: w281 -> [_ w309]
                  frame Default {
                  }
                  frame "MultiRecord" {
                    n98 = Bundle By Name(cluster=T9 {"EncoderReadout States"=enum."SetPointsNum", "Variant"=variant}, "Variant"=w309) -> (w312:T9)
                    n99 = Enqueue Element(queue=w310, element=w312) -> ()  [unwired: 2 in, 3 out]
                  }
                }
                n100 = Less Than 0?(x=w285) -> (x < 0?=w291:bool)
                n101 = Bundle By Name(cluster=w288, "status"=w291, "source"=w284) -> (w296:errorcluster)
              }
              frame Error {
                n102 = xnode "Error Ring"() -> ("error out"=w321:errorcluster)
              }
            }
            n103 = Select(t=w266, s=w265, f=w267) -> (s? t:f=w268:T14)
            n104 = Bundle By Name(cluster=w275, "Acquisition"=w268) -> (w277:T6)
          }
          frame "SetChannels_" {
            n105 = Unbundle By Name(w328) -> ("Channels"=w336:T16)
            n106 = Variant To Data(error in=w333, type=w336, Variant=w337) -> (data=w335:T16, error out=w332:errorcluster)
            n107 = case shown="No Error" w332 {
              selector: w332 -> [w352 _]
              tunnel: w338 -> [w354 _]
              tunnel: w335 -> [w341 _]
              tunnel: [w351 w375] -> w334
              tunnel: w329 -> [w348 _]
              tunnel: w328 -> [w343 w374]
              tunnel: [w342 w374] -> w327
              frame No Error {
                n108 = Bundle By Name(cluster=w343, "Channels"=w341) -> (w342:T6)
                n109 = call <instrlib>:"CleanupDAQTasks.vi"("error in (no error)"=w352, "Queue in"=w348) -> ("error out"=w349:errorcluster)  [unwired: 8 in, 1 out]
                n110 = for {
                  tunnel: w341 -> [w363] mode=indexing
                  shift-right: [w373] -> w353
                  shift-left: w349 -> [w373]
                  tunnel: [w362] -> w347 mode=indexing
                  n111 = Unbundle By Name(w363) -> ("Coupling"=w366:u16, "Differential Input"=w364:bool, "Direct-to-ADC"=w367:bool, "Range"=w368:u32, "Impedance"=w369:u32, "DC Offset"=w370:i32, "Filter"=w371:i32)
                  n112 = Index Array(array=string[] ["DC", "AC"] ("Strings []"), index=w366) -> (element=w365:string)
                  n113 = Bundle(w365, "Differential Input"=w364, "Direct-to-ADC"=w367, "Range"=w368, "Impedance"=w369, "DC Offset"=w370, "Filter"=w371) -> (w362:T17)  [unwired: 1 in]
                }
                n114 = Unbundle By Name(w354) -> ("Handle"=w350:T13)
                n115 = flat-sequence {
                  tunnel: w350 -> [w355]
                  tunnel: [w355] -> w345
                  tunnel: w345 -> [w357]
                  tunnel: [w357] -> w344
                  tunnel: w347 -> [w360]
                  tunnel: w344 -> [w359]
                  tunnel: [w358] -> w346
                  frame #0 {
                    n116 = call <instrlib>:"CsTool-AbortCapture.vi"("Handle Cluster"=w355) -> ()  [unwired: 1 out]
                  }
                  frame #1 {
                    n117 = Wait (ms)(milliseconds to wait=u32 5) -> ()  [unwired: 1 out]
                  }
                  frame #2 {
                    n118 = call <instrlib>:"CsTool-ConfigureChannelArray.vi"("Channels"=w360, "Handle Cluster"=w359) -> ("Error Code"=w361:u32)
                    n119 = call <instrlib>:"CsTool-ErrorHandler.vi"("Error Code"=w361, "Handle Cluster"=w359) -> ("Error String"=w358:string)  [unwired: 1 in]
                  }
                }
                n120 = Bundle By Name(cluster=w353, "source"=w346) -> (w351:errorcluster)
              }
              frame Error {
                n121 = xnode "Error Ring"() -> ("error out"=w375:errorcluster)
              }
            }
          }
          frame "SetTrigger_" {
            n122 = Unbundle By Name(w382) -> ("Trigger"=w390:T18)
            n123 = Variant To Data(error in=w387, type=w390, Variant=w391) -> (data=w389:T18, error out=w386:errorcluster)
            n124 = case shown="No Error" w386 {
              selector: w386 -> [w421 _]
              tunnel: w392 -> [w422 _]
              tunnel: w389 -> [w395 _]
              tunnel: [w405 w432] -> w388
              tunnel: w383 -> [w402 _]
              tunnel: w382 -> [w397 w431]
              tunnel: [w396 w431] -> w381
              frame No Error {
                n125 = Bundle By Name(cluster=w397, "Trigger"=w395) -> (w396:T6)
                n126 = call <instrlib>:"CleanupDAQTasks.vi"("error in (no error)"=w421, "Queue in"=w402) -> ("error out"=w403:errorcluster)  [unwired: 8 in, 1 out]
                n127 = Unbundle By Name(w395) -> ("Slope"=w411:u16, "Level"=w417:i32, "Source"=w416:i32, "External Range"=w415:u32, "External Coupling"=w410:u16, "External"=w420:bool, "Disable"=w419:bool, "External Impedance"=w409:u16)
                n128 = Unbundle By Name(w422) -> ("Handle"=w404:T13)
                n129 = Index Array(array=string[] ["Rising", "Falling"] ("Strings [] 3"), index=w411) -> (element=w408:string)
                n130 = Index Array(array=string[] ["DC", "AC"] ("Strings [] 2"), index=w410) -> (element=w407:string)
                n131 = Index Array(array=string[] ["50 Ohm", "HiZ"] ("Strings []"), index=w409) -> (element=w406:string)
                n132 = flat-sequence {
                  tunnel: w404 -> [w423]
                  tunnel: [w423] -> w399
                  tunnel: w399 -> [w425]
                  tunnel: [w425] -> w398
                  tunnel: w401 -> [w429]
                  tunnel: w398 -> [w427]
                  tunnel: [w428] -> w400
                  frame #0 {
                    n133 = call <instrlib>:"CsTool-AbortCapture.vi"("Handle Cluster"=w423) -> ()  [unwired: 1 out]
                  }
                  frame #1 {
                    n134 = Wait (ms)(milliseconds to wait=u32 5) -> ()  [unwired: 1 out]
                  }
                  frame #2 {
                    n135 = call <instrlib>:"CsTool-ConfigureTriggerArray.vi"("Triggers"=w429, "Handle Cluster"=w427) -> ("Error Code"=w430:i32)
                    n136 = call <instrlib>:"CsTool-ErrorHandler.vi"("StopOnError (true)"=FALSE, "Error Code"=w430, "Handle Cluster"=w427) -> ("Error String"=w428:string)
                  }
                }
                n137 = Bundle(w408, "Level"=w417, "Source"=w416, "External Range"=w415, w407, "External"=w420, "Disable"=w419, w406) -> (w418:T19)  [unwired: 1 in]
                n138 = Build Array(w418) -> (w401:T20)
                n139 = Bundle By Name(cluster=w403, "source"=w400) -> (w405:errorcluster)
              }
              frame Error {
                n140 = xnode "Error Ring"() -> ("error out"=w432:errorcluster)
              }
            }
          }
          frame "SetSegment#_" {
            n141 = Unbundle By Name(w449) -> ("Acquisition"=w441:T14)
            n142 = Variant To Data(error in=w448, type=u32 1 ("Segment Count (1)"), Variant=w450) -> (data=w439:u32, error out=w447:errorcluster)
            n143 = case shown="No Error" w447 {
              selector: w447 -> [w473 _]
              tunnel: w452 -> [w483 _]
              tunnel: w441 -> [w456 w496]
              tunnel: [w472 w497] -> w442
              tunnel: w444 -> [w466 _]
              tunnel: w443 -> [w463 _]
              tunnel: [w457 w496] -> w438
              tunnel: w439 -> [w455 _]
              frame No Error {
                n144 = call <instrlib>:"CleanupDAQTasks.vi"("error in (no error)"=w473, "Queue in"=w463) -> ("error out"=w464:errorcluster)  [unwired: 8 in, 1 out]
                n145 = Unbundle By Name(w456) -> ("Mode"=w469:u16, "Sample Rate"=w482:dbl, "Clock mode"=w481:enum16{"Internal", "External", "Reference"})
                n146 = Unbundle By Name(w456) -> ("Depth"=w474:dbl, "Segment Size"=w480:dbl, "Trigger Timeout"=w479:dbl, "Trigger Holdoff"=w478:dbl, "Trigger Delay"=w477:dbl)
                n147 = Unbundle By Name(w483) -> ("Handle"=w471:T13, "Mode(Gage)"=w465:T12)
                n148 = Index Array(array=string[] ["Single", "Dual", "Quad", "Octal"], index=w469) -> (element=w475:string)
                n149 = Scale By Power Of 2(n=w469, x=ext 1.0) -> (x*2^n=w470:ext)
                n150 = To Long Integer(number=w470) -> ()  [unwired: 1 out]
                n151 = Bundle("Sample Rate"=w482, "Clock mode"=w481, w475, "Depth"=w474, "Segment Size"=w480, "Trigger Timeout"=w479, "Trigger Holdoff"=w478, "Trigger Delay"=w477) -> (w462:T15)  [unwired: 1 in]
                n152 = To Long Integer(number=w474) -> ()  [unwired: 1 out]
                n153 = flat-sequence {
                  tunnel: w471 -> [w488]
                  tunnel: [w488] -> w459
                  tunnel: w459 -> [w490]
                  tunnel: [w490] -> w458
                  tunnel: w458 -> [w495]
                  tunnel: w462 -> [w494]
                  tunnel: [w493] -> w461
                  tunnel: [w492] -> w460
                  tunnel: w455 -> [w491]
                  frame #0 {
                    n154 = call <instrlib>:"CsTool-AbortCapture.vi"("Handle Cluster"=w488) -> ()  [unwired: 1 out]
                  }
                  frame #1 {
                    n155 = Wait (ms)(milliseconds to wait=u32 5) -> ()  [unwired: 1 out]
                  }
                  frame #2 {
                    n156 = call <instrlib>:"CsTool-ConfigureAcquisition.vi"("Handle Cluster"=w495, "Segment Count (1)"=w491, "Acquisition"=w494) -> ("Error Code"=w493:i32)  [unwired: 2 in]
                    n157 = call <instrlib>:"CsTool-ErrorHandler.vi"("Error Code"=w493, "Handle Cluster"=w495) -> ("Error String"=w492:string)  [unwired: 1 in]
                  }
                }
                n158 = case shown="\"MultiRecord\"" w465 {
                  tunnel: w466 -> [_ w485]
                  tunnel: w455 -> [_ w484]
                  frame Default {
                  }
                  frame "MultiRecord" {
                    n159 = Bundle By Name(cluster=T9 {"EncoderReadout States"=enum."SetPointsNum", "Variant"=variant}, "Variant"=w484) -> (w487:T9)
                    n160 = Enqueue Element(queue=w485, element=w487) -> ()  [unwired: 2 in, 3 out]
                  }
                }
                n161 = Less Than 0?(x=w461) -> (x < 0?=w467:bool)
                n162 = Bundle By Name(cluster=w464, "status"=w467, "source"=w460) -> (w472:errorcluster)
                n163 = Bundle By Name(cluster=w456, "Segment"=w455) -> (w457:T14)
                "Segment Count (1)" <- w455
              }
              frame Error {
                n164 = xnode "Error Ring"() -> ("error out"=w497:errorcluster)
              }
            }
            n165 = Bundle By Name(cluster=w449, "Acquisition"=w438) -> (w451:T6)
          }
          frame "SetAll_AcquChTrig_" {
            n166 = Variant To Data(type=w509, Variant=w510) -> (data=w507:T6, error out=w508:errorcluster)  [unwired: 1 in]
            n167 = case shown="No Error" w508 {
              tunnel: w512 -> [w532 _]
              tunnel: [w531 w537] -> w511
              tunnel: w507 -> [w530 _]
              tunnel: w506 -> [w529 _]
              frame No Error {
                n168 = Unbundle By Name(w530) -> ("Mode(Gage)"=w519:T12, "Acquisition"=w527:T14, "Channels"=w525:T16, "Trigger"=w523:T18)
                n169 = Bundle By Name(cluster=T3 {"GenericDAQ State"=enum."SetMode_", "Variant"=variant} ("element"), "Variant"=w519) -> (w516:T3)
                n170 = Bundle By Name(cluster=T3 {"GenericDAQ State"=enum."SetAcquisition_", "Variant"=variant} ("element"), "Variant"=w527) -> (w517:T3)
                n171 = Bundle By Name(cluster=T3 {"GenericDAQ State"=enum."SetChannels_", "Variant"=variant} ("element"), "Variant"=w525) -> (w515:T3)
                n172 = Bundle By Name(cluster=T3 {"GenericDAQ State"=enum."SetTrigger_", "Variant"=variant} ("element"), "Variant"=w523) -> (w522:T3)
                n173 = Build Array(w516, w517, w515, w522) -> (w521:T3[])
                n174 = Reverse 1D Array(array=w521) -> (reversed array=w518:T3[])
                n175 = for "Has to be at the \nopposite end, otherwise\nrace condition" {
                  tunnel: w532 -> [w536]
                  shift-right: [w535] -> w531
                  shift-left: w529 -> [w534]
                  tunnel: w518 -> [w533] mode=indexing
                  n176 = Enqueue Element At Opposite End(queue=w536, element=w533, error in (no error)=w534) -> (error out=w535:errorcluster)  [unwired: 1 in, 2 out]
                }
              }
              frame Error {
                n177 = xnode "Error Ring"() -> ("error out"=w537:errorcluster)
              }
            }
          }
          frame "fConfigurate" {
            # "If dependancy of ErrorLog missing, \njust remove errorlog vi."
            # "fConfigurate => Commit (as in Gage SDK)"
            n178 = Unbundle By Name(w555) -> ("Handle"=w554:T13)
            n179 = call <instrlib>:"CleanupDAQTasks.vi"("error in (no error)"=w548, "Queue in"=w543) -> ("error out"=w544:errorcluster)  [unwired: 8 in, 1 out]
            n180 = flat-sequence {
              tunnel: w554 -> [w559]
              tunnel: [w559] -> w551
              tunnel: w551 -> [w562]
              tunnel: [w563] -> w549
              tunnel: [w561] -> w545
              frame #0 {
                n181 = disable-structure shown="Enabled" {
                  disable-tunnel: w559 -> [w560 _]
                  frame Disabled {
                    n182 = call <instrlib>:"CsTool-AbortCapture.vi"("Handle Cluster"=w560) -> ()  [unwired: 1 out]
                  }
                  frame Enabled {
                  }
                }
              }
              frame #1 {
                n183 = call <instrlib>:"CsTool-Commit.vi"("Handle Cluster"=w562) -> ("Error Code"=w561:i32)  [unwired: 2 in, 1 out]
                n184 = call <instrlib>:"CsTool-ErrorHandler.vi"("StopOnError (true)"=FALSE, "Error Code"=w561, "Handle Cluster"=w562) -> ("Error String"=w563:string)
                n185 = case shown="True" FALSE {
                  tunnel: w562 -> [_ w567]
                  tunnel: w561 -> [_ w566]
                  frame False {
                  }
                  frame True {
                    n186 = call <instrlib>:"DisplayCurrentConfiguration.vi"("error code  in"=w566, "Handle Cluster"=w567) -> ()  [unwired: 10 in]
                  }
                }
              }
            }
            n187 = Less Than 0?(x=w545) -> (x < 0?=w547:bool)
            n188 = Bundle By Name(cluster=w544, "code"=w545, "status"=w547, "source"=w549) -> (w550:errorcluster)
            n189 = call <userlib>:"ErrorLog.vi"("error in (no error)"=w550) -> ("error out"=w546:errorcluster)  [unwired: 10 in]
          }
          frame "fStart" {
            # "Must ensure that laser is not firing here"
            # "Known issue:\n\nIf too manu fStart send here, virtual system crash.\nhas to restart Lv"
            # "Prevent program termination, \nwhen capture executed \nbefore previous one finished\n\nCould not find how to detect\na unfinished capture\n\nIn GetDate frame, capture actions is \nguarentted finished, no need to do so."
            n190 = Unbundle By Name(w579) -> ("Handle"=w584:T13, "Mode(Gage)"=w580:T12)
            n191 = Unbundle By Name(w579) -> ("SecondaryDataVIRef"=w578:refnum<vi>, "Option(SecondaryDataVI)"=w577:i32)
            n192 = call <instrlib>:"CleanupDAQTasks.vi"("error in (no error)"=w575, "Queue in"=w573) -> ("error out"=w574:errorcluster, "Queue out"=w572:refnum<queue>)  [unwired: 8 in]
            n193 = Enqueue Element(queue=w572, element=T3 {"GenericDAQ State"=enum."_WaitForDone/Idle", "Variant"=variant}, error in (no error)=w574) -> (error out=w587:errorcluster)  [unwired: 1 in, 2 out]
            n194 = case shown="\"MultiRecord\"" w580 {
              tunnel: w581 -> [_ w599]
              tunnel: w578 -> [_ w597]
              tunnel: w577 -> [_ w598]
              tunnel: w576 -> [_ _]
              tunnel: w569 -> [_ w595]
              tunnel: [_ w592] -> w568
              frame Default {
              }
              frame "MultiRecord" {
                n195 = Not A Number/Path/Refnum?(number/path/refnum=w597) -> (NaN/Path/Refnum?=w596:bool)
                n196 = disable-structure shown="Disabled" {
                  disable-tunnel: [w620 w630 w632] -> w594
                  disable-tunnel: w599 -> [w619 w629 w632]
                  disable-tunnel: w598 -> [w618 _ _]
                  disable-tunnel: w597 -> [w617 _ _]
                  disable-tunnel: w596 -> [w616 _ _]
                  frame Disabled {
                    n197 = case shown="False" w616 {
                      tunnel: [w627 w628] -> w620
                      tunnel: w619 -> [w624 w628]
                      tunnel: w617 -> [w623 _]
                      tunnel: w618 -> [w622 _]
                      frame False {
                        n198 = call-by-ref "?"(reference=w623, "Option"=w622) -> ("SecondaryData"=w621:dbl[])  [unwired: 11 in, 2 out]
                        n199 = Bundle By Name(cluster=T9 {"EncoderReadout States"=enum."SetPosition", "Variant"=variant}, "Variant"=w621) -> (w625:T9)
                        n200 = Enqueue Element(queue=w624, element=w625) -> (queue out=w627:refnum<queue>)  [unwired: 2 in, 2 out]
                      }
                      frame True {
                      }
                    }
                  }
                  frame Disabled {
                    n201 = Enqueue Element(queue=w629, element=T9 {"EncoderReadout States"=enum."FlushBuffer", "Variant"=variant}) -> (queue out=w630:refnum<queue>)  [unwired: 2 in, 2 out]
                  }
                  frame Enabled {
                  }
                }
                n202 = disable-structure shown="Enabled" {
                  disable-tunnel: w594 -> [w614 _]
                  disable-tunnel: w595 -> [w612 _]
                  disable-tunnel: [w610 _] -> _
                  disable-tunnel: [w609 _] -> w593
                  frame Enabled {
                    n203 = Bundle By Name(cluster=T9 {"EncoderReadout States"=enum."QueryStatus", "Variant"=variant}, "Variant"=w612) -> (w613:T9)
                    n204 = Enqueue Element(queue=w614, element=w613) -> (queue out=w609:refnum<queue>, error out=w611:errorcluster)  [unwired: 2 in, 1 out]
                    n205 = Dequeue Element(queue=w612, error in (no error)=w611) -> (element=→"element":T1, error out=w610:errorcluster)  [unwired: 1 in, 2 out]
                  }
                  frame Disabled {
                  }
                }
                n206 = disable-structure shown="Enabled" {
                  disable-tunnel: w593 -> [w602 w605 w607]
                  disable-tunnel: [w601 w604 w607] -> _
                  disable-tunnel: [w600 _ _] -> w592
                  frame Enabled {
                    n207 = Enqueue Element(queue=w602, element=T9 {"EncoderReadout States"=enum."GetPositions", "Variant"=variant}) -> (queue out=w601:refnum<queue>, error out=w600:errorcluster)  [unwired: 2 in, 1 out]
                  }
                  frame Disabled {
                    n208 = Enqueue Element(queue=w605, element=T9 {"EncoderReadout States"=enum."Start(Flush)", "Variant"=variant}) -> (queue out=w604:refnum<queue>)  [unwired: 2 in, 2 out]
                  }
                  frame Disabled {
                  }
                }
              }
            }
            n209 = flat-sequence {
              tunnel: w584 -> [w633]
              tunnel: [w633] -> w571
              tunnel: w571 -> [w635]
              tunnel: [w635] -> w570
              tunnel: w570 -> [w637]
              tunnel: [w636] -> w582
              tunnel: w568 -> [_]
              frame #0 {
                n210 = call <instrlib>:"CsTool-AbortCapture.vi"("Handle Cluster"=w633) -> ()  [unwired: 1 out]
              }
              frame #1 {
                n211 = Wait (ms) "Prevent crash if too many \nfStart sent in short time."(milliseconds to wait=u32 50) -> ()  [unwired: 1 out]
              }
              frame #2 {
                n212 = call <instrlib>:"CsTool-Capture.vi"("Handle Cluster"=w637) -> ("Error Code"=w638:i32)
                n213 = call <instrlib>:"CsTool-ErrorHandler.vi"("Error Code"=w638, "Handle Cluster"=w637) -> ("Error String"=w636:string)  [unwired: 1 in]
              }
            }
            n214 = Bundle By Name(cluster=w587, "source"=w582) -> (w583:errorcluster)
          }
          frame "GetStatus" {
            n215 = Unbundle By Name(w640) -> ("Handle"=w641:T13)
            n216 = call <instrlib>:"CsTool-QueryStatus.vi"("Handle Cluster"=w641) -> ("Status"=w639:i32)
            n217 = Bundle By Name(cluster=w640, "DAQ_Status"=w639) -> (w644:T4)
          }
          frame "_WaitForDone/Idle" {
            w663 = T2[] [enum."Close", enum."CloseAll", enum."Reset", enum."Quit", enum."Abort"] items=["Enumerate", "Open", "Close", "CloseAll", "Reset", "Quit", "==Settings==", "SetAcquisition_", "SetChannels_", "SetTrigger_", "SetAnalogTrigDetector_", "SetSegment#_", "SetAll_AcquChTrig_", "fConfigurate", "fStart", "GetStatus", "_WaitForDone/Idle", "_GetData", "GetAcquisition", "GetChannels", "GetTrigger", "GetAll_AcquChTrig", "Abort", "==Messaging==", "_PushDataOut", "GetStat_", "GetConfig_", "==ModeSetup==", "SetSignalBuffer_", "SetMode_", "SetSecondaryDataRef._", "SetDynamicBuffer_", "==AnalogOut==", "GetChannelCount_AO", "fStart_AO", "SetChEnable_AO", "SetConfig_AO", "SetFuncData_AO", "SetOffset_AO_", "SetMasterNode_AO", "SetStates_AO", "SetSymetry_AO", "SetTriggerSource_AO", "==Trigger==", "ManualTrigger", "===Sync===", "LineStart", "LineEnd", "FrameStart", "FrameEnd", "EOL_PassThrough", "SOL_PassThrough"]
            # "to be considered \n\nwhat if system not configed??\nwhat status is that?"
            # "0 dne\n1 armed\n2 triggered\n3 transfering"
            n218 = Unbundle By Name(w668) -> ("Mode(Gage)"=w652:T12, "Handle"=w658:T13)
            n219 = call <instrlib>:"CsTool-QueryStatus.vi"("Handle Cluster"=w658) -> ("Status"=w655:i32)
            n220 = Bundle By Name(cluster=w668, "DAQ_Status"=w655) -> (w667:T4)
            n221 = Preview Queue Element(queue=w676, timeout in ms (-1)=0, error in (no error)=w675) -> (queue out=w671:refnum<queue>, element=w665:T3, timed out?=w664:bool, error out=w670:errorcluster)
            n222 = Unbundle(w665) -> ("GenericDAQ State"=w660:T2)  [unwired: 1 out]
            n223 = Search 1D Array(1D array=w663, element=w660) -> (index of element=w662:i32)  [unwired: 1 in]
            n224 = Equal?(x=T12."MultiRecord", y=w652) -> (x = y?=w650:bool)
            n225 = Greater Or Equal To 0?(x=w662) -> (x >= 0?=w661:bool)
            n226 = Select "Lower CPU consumption \nin MultiRecord Mode"(t=u32 500 ("milliseconds to wait"), s=w650, f=u32 0) -> (s? t:f=w653:u32)
            n227 = Compound Arithmetic op=AND(w661, invert w664) -> (w659:bool)
            n228 = case shown="False" w659 {
              tunnel: w671 -> [w680 _]
              tunnel: w670 -> [w679 w697]
              tunnel: [w678 w697] -> w669
              tunnel: w655 -> [w677 _]
              frame False {
                n229 = case shown="2, Default" w677 {
                  tunnel: w680 -> [w681 w692 w696]
                  tunnel: w679 -> [w684 w691 w695]
                  tunnel: [w683 w690 w694] -> w678
                  frame 1 {
                    # "armed ??"
                    # "Typically, this is caused by config change\nduring acquisition. \nPush fConfig and fStart to continure  acuisition."
                    # "armed, not configed??"
                    n230 = for {
                      shift-right: [w687] -> w683
                      shift-left: w684 -> [w688]
                      tunnel: T3[] [{"GenericDAQ State"=enum."_WaitForDone/Idle", "Variant"=variant}] -> [w686] mode=indexing
                      tunnel: w681 -> [w685]
                      n231 = Enqueue Element(queue=w685, element=w686, error in (no error)=w688) -> (error out=w687:errorcluster)  [unwired: 1 in, 2 out]
                    }
                  }
                  frame 0 {
                    # "Done"
                    n232 = Enqueue Element(queue=w692, element=T3 {"GenericDAQ State"=enum."_GetData", "Variant"=variant}, error in (no error)=w691) -> (error out=w690:errorcluster)  [unwired: 1 in, 2 out]
                  }
                  frame 2, Default {
                    # "triggered"
                    # "triggered, others"
                    n233 = Enqueue Element(queue=w696, element=T3 {"GenericDAQ State"=enum."_WaitForDone/Idle", "Variant"=variant}, error in (no error)=w695) -> (error out=w694:errorcluster)  [unwired: 1 in, 2 out]
                  }
                }
              }
              frame True {
              }
            }
            n234 = Wait (ms)(milliseconds to wait=w653) -> ()  [unwired: 1 out]
          }
          frame "_GetData" {
            n235 = Unbundle By Name(w730) -> ("Acquisition.Segment"=w710:u32, "Channels"=w720:T16, "Acquisition.Depth"=w699:dbl, "Acquisition.Start (0)"=w700:dbl)
            n236 = Unbundle By Name(w722) -> ("TrigCount"=w721:i32, "Option(SecondaryDataVI)"=w718:i32, "SecondaryDataVIRef"=w719:refnum<vi>, "Handle"=w712:T13)
            n237 = Unbundle By Name(w722) -> ("Mode(Gage)"=w709:T12)
            n238 = Enqueue Element(queue=w726, element=T3 {"GenericDAQ State"=enum."_PushDataOut", "Variant"=variant}, error in (no error)=w724) -> (queue out=w708:refnum<queue>, error out=w715:errorcluster)  [unwired: 1 in, 1 out]
            n239 = Array Size(array=w720) -> (size(s)=w707:i32)
            n240 = To Long Integer(number=w710) -> (32bit integer=w698:i32)
            n241 = Add(x=w721, y=w698) -> (x+y=w723:i32)
            n242 = Bundle By Name(cluster=w722, "TrigCount"=w723) -> (w717:T4)
            n243 = case shown="\"MultiRecord\"" w709 {
              tunnel: w728 -> [w780 w790]
              tunnel: [w779 w790] -> w727
              tunnel: [w775 w785] -> w714
              tunnel: w712 -> [w771 w784]
              tunnel: w719 -> [w778 _]
              tunnel: w718 -> [w777 _]
              tunnel: w715 -> [w775 w785]
              tunnel: w717 -> [w772 w789]
              tunnel: [w772 w788] -> w716
              tunnel: w710 -> [_ w786]
              tunnel: [w771 w784] -> w706
              frame Default {
                n244 = Not A Number/Path/Refnum?(number/path/refnum=w778) -> (NaN/Path/Refnum?=w773:bool)
                n245 = case shown="True" w773 {
                  tunnel: [w783 _] -> w774
                  tunnel: w778 -> [w782 _]
                  tunnel: w777 -> [w781 _]
                  frame False {
                    n246 = call-by-ref "?"(reference=w782, "Option"=w781) -> ("SecondaryData"=w783:dbl[])  [unwired: 11 in, 2 out]
                  }
                  frame True {
                  }
                }
                n247 = Tick Count (ms)() -> (millisecond timer value=w776:u32)
                n248 = Bundle By Name(cluster=w780, "tickcount"=w776, "SecondaryData"=w774) -> (w779:T10)
              }
              frame "MultiRecord" {
                n249 = call <instrlib>:"CsTool-TransferTimeStamp.vi"("Length (1)"=w786, "Handle Cluster"=w784) -> ("TS Time"=w787:dbl[])  [unwired: 1 in, 2 out]
                n250 = Bundle By Name(cluster=w789, "TSArray"=w787) -> (w788:T4)
              }
            }
            n251 = case shown="\"MultiRecord\"" w709 {
              tunnel: w714 -> [w734 w745 w753 w755]
              tunnel: [w734 w744 w753 w754] -> w713
              tunnel: w708 -> [_ _ _ w756]
              tunnel: w707 -> [_ _ _ w760]
              tunnel: w706 -> [_ w736 w747 w761]
              tunnel: w705 -> [w732 w741 w752 w763]
              tunnel: w704 -> [w731 w740 w751 w762]
              tunnel: [w732 w739 w750 w759] -> w703
              tunnel: [w731 w738 w749 w758] -> w702
              tunnel: [w733 w735 w746 w757] -> w701
              tunnel: w700 -> [_ w737 w748 _]
              tunnel: w699 -> [w733 w735 w746 _]
              frame Default {
              }
              frame "Continuous" {
                n252 = call "GageTransfer-SingleRec_Mod.vi"("Handle Cluster"=w736, "Start (0)"=w737, "Length (4096)"=w735, "Buffer in I16"=w741, "Buffer in U8"=w740) -> ("Buffer Out I16"=w739:i16[], "Buffer Out U8"=w738:u8[])  [unwired: 7 in, 2 out]
                n253 = call <instrlib>:"CsTool-Capture.vi"("Handle Cluster"=w736) -> ("Error Code"=w743:i32)
                n254 = call <instrlib>:"CsTool-ErrorHandler.vi"("Error Code"=w743, "Handle Cluster"=w736) -> ("Error String"=w742:string)  [unwired: 1 in]
                n255 = Bundle By Name(cluster=w745, "source"=w742) -> (w744:errorcluster)
              }
              frame "Normal" {
                n256 = call "GageTransfer-SingleRec_Mod.vi"("Handle Cluster"=w747, "Start (0)"=w748, "Length (4096)"=w746, "Buffer in I16"=w752, "Buffer in U8"=w751) -> ("Buffer Out I16"=w750:i16[], "Buffer Out U8"=w749:u8[])  [unwired: 7 in, 2 out]
              }
              frame "MultiRecord" {
                w764 = u32 64  # tail length: CobraMax: 64
                n257 = disable-structure shown="Enabled" {
                  disable-tunnel: w756 -> [w768 _]
                  disable-tunnel: w755 -> [w767 w770]
                  disable-tunnel: [w766 w770] -> w754
                  frame Enabled {
                    n258 = Enqueue Element(queue=w768, element=T3 {"GenericDAQ State"=enum."fStart", "Variant"=variant}, error in (no error)=w767) -> (error out=w766:errorcluster)  [unwired: 1 in, 2 out]
                  }
                  frame Disabled {
                  }
                }
                n259 = call "GageTransfer-AdvMultiRec_Hack.vi"("Handle Cluster"=w761, "Channels"=w760, "tail ength"=w764, "Buffer in I16"=w763, "Buffer in U8"=w762) -> ("Buffer Out I16"=w759:i16[], "Buffer Out U8"=w758:u8[], "elapsed time(ms)"=→"transfer time":u32, "Adj.SegmentSize"=w757:dbl)  [unwired: 4 in, 3 out]
              }
            }
            n260 = Bundle By Name(cluster=w716, "Adj.SegmenttSize"=w701) -> (w711:T4)
          }
          frame "GetAcquisition" {
            # "Mode and Segment Count"
            n261 = Unbundle By Name(w810) -> ("Handle"=w794:T13)
            n262 = call <instrlib>:"CsTool-QueryAcquisitionParameters.vi"("Handle Cluster"=w794) -> ("Error Code"=w793:i32, "Trigger Holdoff"=w808:dbl, "Trigger Delay"=w807:dbl, "Output Handle Cluster"=w804:T21, "Sample Rate"=w806:dbl, "Clock Mode"=w803:enum16{"Internal", "External", "Reference"}, "Mode"=w796:string, "Trigger Timeout"=w800:dbl, "Segment Size"=w801:dbl, "Depth"=w802:dbl)  [unwired: 4 in, 1 out]
            n263 = call <instrlib>:"CsTool-ErrorHandler.vi"("Error Code"=w793, "Handle Cluster"=w794) -> ("Error String"=w791:string)  [unwired: 1 in]
            n264 = Bundle By Name(cluster=w813, "source"=w791) -> (w792:errorcluster)
            n265 = Bundle By Name(cluster=w810, "Handle"=w804) -> (w805:T4)
            n266 = Search 1D Array(1D array=string[] ["Single", "Dual", "Quad", "Octal"], element=w796) -> (index of element=w795:i32)  [unwired: 1 in]
            n267 = Bundle By Name(cluster=w811, "Acquisition.Sample Rate"=w806, "Acquisition.Mode"=w795, "Acquisition.Depth"=w802, "Acquisition.Segment Size"=w801, "Acquisition.Trigger Timeout"=w800, "Acquisition.Trigger Holdoff"=w808, "Acquisition.Trigger Delay"=w807, "Acquisition.Clock mode"=w803) -> (w809:T6)
          }
          frame "GetChannels" {
            n268 = Unbundle By Name(w823) -> ("Handle"=w825:T13)
            n269 = Unbundle By Name(w822) -> ("Channels"=w821:T16)
            n270 = for {
              tunnel: w825 -> [w830]
              tunnel: w821 -> [w842] mode=indexing
              tunnel: [w835] -> w820 mode=indexing
              tunnel: [w829] -> w816 mode=indexing
              i -> [w843]
              n271 = call <instrlib>:"CsTool-QueryChannelParameters.vi"("Handle Cluster"=w830, "Channel"=w843) -> ("Filter"=w836:u32, "Coupling"=w833:string, "Differential Input"=w841:bool, "Direct-to-ADC"=w837:bool, "Range (mV)"=w840:u32, "Impedance"=w839:u32, "DC Offset (mV)"=w838:u32, "Error Code"=w831:i32)
              n272 = call <instrlib>:"CsTool-ErrorHandler.vi"("Error Code"=w831, "Handle Cluster"=w830) -> ("Error String"=w829:string)  [unwired: 1 in]
              n273 = Search 1D Array(1D array=string[] ["DC", "AC"], element=w833) -> (index of element=w832:i32)  [unwired: 1 in]
              n274 = Bundle By Name(cluster=w842, "Differential Input"=w841, "Range"=w840, "Impedance"=w839, "DC Offset"=w838, "Direct-to-ADC"=w837, "Coupling"=w832, "Filter"=w836) -> (w835:T22)
            }
            n275 = Concatenate Strings(w816) -> (w815:string)
            n276 = Bundle By Name(cluster=w822, "Channels"=w820) -> (w824:T6)
            n277 = Bundle By Name(cluster=w827, "source"=w815) -> (w817:errorcluster)
          }
          frame "GetTrigger" {
            n278 = Unbundle By Name(w864) -> ("Handle"=w846:T13)
            n279 = call <instrlib>:"CsTool-QueryTriggerParameters.vi"("Handle Cluster"=w846, "Trigger"=u32 0) -> ("External Impedance"=w850:string, "External Range (mV)"=w862:u32, "External Coupling"=w853:string, "Error Code"=w847:i32, "Source"=w861:i32, "Slope"=w856:string, "Level"=w860:i32, "External Trigger"=w859:bool, "Disable Trigger"=w858:bool)  [unwired: 9 in]
            n280 = call <instrlib>:"CsTool-ErrorHandler.vi"("Error Code"=w847, "Handle Cluster"=w846) -> ("Error String"=w844:string)  [unwired: 1 in]
            n281 = Search 1D Array(1D array=string[] ["rising", "falling"], element=w856) -> (index of element=w855:i32)  [unwired: 1 in]
            n282 = Search 1D Array(1D array=string[] ["dc", "ac"], element=w853) -> (index of element=w852:i32)  [unwired: 1 in]
            n283 = Search 1D Array(1D array=string[] ["50 Ohm", "HiZ"], element=w850) -> (index of element=w849:i32)  [unwired: 1 in]
            n284 = Bundle By Name(cluster=w869, "source"=w844) -> (w845:errorcluster)
            n285 = Bundle By Name(cluster=w868, "Trigger.External Range"=w862, "Trigger.Source"=w861, "Trigger.Slope"=w855, "Trigger.Level"=w860, "Trigger.External"=w859, "Trigger.Disable"=w858, "Trigger.External Coupling"=w852, "Trigger.External Impedance"=w849) -> (w863:T6)
          }
          frame "GetAll_AcquChTrig" {
            n286 = for "Has to be at the \nopposite end, otherwise\nrace condition" {
              tunnel: w874 -> [w884]
              shift-right: [w883] -> w872
              shift-left: w873 -> [w882]
              tunnel: T3[] [{"GenericDAQ State"=enum."GetAcquisition", "Variant"=variant}, {"GenericDAQ State"=enum."GetChannels", "Variant"=variant}, {"GenericDAQ State"=enum."GetTrigger", "Variant"=variant}] -> [w881] mode=indexing
              n287 = Enqueue Element At Opposite End(queue=w884, element=w881, error in (no error)=w882) -> (error out=w883:errorcluster)  [unwired: 1 in, 2 out]
            }
          }
          frame "Abort" {
            n288 = Unbundle By Name(w892) -> ("Handle"=w895:T13, "Mode(Gage)"=w893:T12)
            n289 = Unbundle By Name(w892) -> ("SecondaryDataVIRef"=w890:refnum<vi>, "Option(SecondaryDataVI)"=w888:i32)
            n290 = call <instrlib>:"CleanupDAQTasks.vi"("error in (no error)"=w897, "Queue in"=w898) -> ("error out"=w896:errorcluster, "Queue out"=w887:refnum<queue>)  [unwired: 8 in]
            n291 = flat-sequence {
              tunnel: w895 -> [w908]
              tunnel: [w907] -> w894
              tunnel: w893 -> [w907]
              tunnel: [w906] -> w891
              tunnel: w890 -> [w906]
              tunnel: [w905] -> w889
              tunnel: w888 -> [w905]
              tunnel: w887 -> [_]
              tunnel: [w904] -> w886
              tunnel: w885 -> [w904]
              tunnel: w894 -> [w912]
              tunnel: w891 -> [w911]
              tunnel: w889 -> [w910]
              tunnel: w886 -> [w909]
              frame #0 {
                n292 = call <instrlib>:"CsTool-AbortCapture.vi"("Handle Cluster"=w908) -> ()  [unwired: 1 out]
              }
              frame #1 {
                n293 = case shown="\"MultiRecord\"" w912 {
                  tunnel: w911 -> [_ w915]
                  tunnel: w910 -> [_ w914]
                  tunnel: w909 -> [_ w913]
                  frame Default {
                  }
                  frame "MultiRecord" {
                    # "Gage Multirecord Abort will be executed each line\nwhile encoder abort will cause position lost.\nHence, encoder aborting should not be done here."
                    n294 = disable-structure shown="Disabled" {
                      disable-tunnel: w915 -> [w918 _ _]
                      disable-tunnel: w914 -> [w917 _ _]
                      disable-tunnel: w913 -> [w916 w929 _]
                      frame Disabled {
                        n295 = Not A Number/Path/Refnum?(number/path/refnum=w918) -> (NaN/Path/Refnum?=w919:bool)
                        n296 = case shown="False" w919 {
                          tunnel: [w926 w927] -> _
                          tunnel: w916 -> [w923 w927]
                          tunnel: w918 -> [w922 _]
                          tunnel: w917 -> [w921 _]
                          frame False {
                            n297 = call-by-ref "?"(reference=w922, "Option"=w921) -> ("SecondaryData"=w920:dbl[])  [unwired: 11 in, 2 out]
                            n298 = Bundle By Name(cluster=T9 {"EncoderReadout States"=enum."SetPosition", "Variant"=variant}, "Variant"=w920) -> (w924:T9)
                            n299 = Enqueue Element(queue=w923, element=w924) -> (queue out=w926:refnum<queue>)  [unwired: 2 in, 2 out]
                          }
                          frame True {
                          }
                        }
                      }
                      frame Disabled {
                        n300 = Enqueue Element(queue=w929, element=T9 {"EncoderReadout States"=enum."Stop", "Variant"=variant}) -> ()  [unwired: 2 in, 3 out]
                      }
                      frame Enabled {
                      }
                    }
                  }
                }
              }
            }
          }
          frame "==Messaging==" {
            # "Invalid Frame"
            n301 = xnode "Error Ring"() -> ("error out"=w932:errorcluster)
          }
          frame "_PushDataOut" {
            # "How to set the timeout??"
            n302 = Unbundle By Name(w972) -> ("Channels"=w960:T16, "Acquisition.Segment"=w952:u32, "Acquisition.Depth"=w959:dbl)
            n303 = Unbundle By Name(w942) -> ("Adj.SegmenttSize"=w955:dbl, "Handle.Offset"=w943:i32, "Handle.Resolution"=w945:i32, "Handle.Sample size"=w944:u32, "TSArray"=w970:dbl[], "SecondaryDataVIRef"=w949:refnum<vi>, "Option(SecondaryDataVI)"=w948:i32, "Mode(Gage)"=w946:T12)
            n304 = Index Array(array=w960) -> (element=w963:T22)  [unwired: 1 in]
            n305 = Unbundle By Name(w963) -> ("DC Offset"=w962:i32, "Range"=w961:u32)
            n306 = Unbundle By Name(w971) -> ()  [unwired: 1 out]
            n307 = Compound Arithmetic op=MULTIPLY(w962, 0.001) -> (w966:dbl)
            n308 = Compound Arithmetic op=MULTIPLY(invert w945, w961, 0.0005) -> (w964:dbl)
            n309 = Multiply(x=w943, y=w964) -> (x*y=w967:dbl)
            n310 = Add(x=w966, y=w967) -> (x+y=w965:dbl)
            n311 = To Single Precision Float(number=w964) -> (single precision float=w958:sgl)
            n312 = To Single Precision Float(number=w965) -> (single precision float=w957:sgl)
            n313 = case shown="\"MultiRecord\"" w946 {
              tunnel: w973 -> [w981 _ w1008 _]
              tunnel: w971 -> [w984 w997 w1034 _]
              tunnel: w970 -> [_ _ w1033 _]
              tunnel: w959 -> [w975 w992 w1032 _]
              tunnel: w958 -> [w987 w1000 w1031 _]
              tunnel: w957 -> [w986 w999 w1030 _]
              tunnel: w956 -> [w985 w998 w1028 _]
              tunnel: w955 -> [_ _ w1024 _]
              tunnel: w954 -> [_ _ w1012 _]
              tunnel: w953 -> [w977 w1003 w1023 w1062]
              tunnel: w952 -> [w980 w995 w1021 _]
              tunnel: [w977 w1003 w1020 w1062] -> w951
              tunnel: w949 -> [_ _ w1019 _]
              tunnel: w948 -> [_ _ w1018 _]
              tunnel: w947 -> [_ _ _ _]
              tunnel: w945 -> [_ _ _ _]
              tunnel: w944 -> [_ _ _ _]
              tunnel: w943 -> [_ _ _ _]
              tunnel: w942 -> [w979 w994 _ _]
              frame "Continuous" {
                # "dont remember why"
                n314 = Enqueue Element(queue=w981, element=T3 {"GenericDAQ State"=enum."_WaitForDone/Idle", "Variant"=variant}) -> ()  [unwired: 2 in, 3 out]
                n315 = Array Subset(array=w977, length=w975) -> (w978:u8[])  [unwired: 1 in]
                n316 = To Single Precision Float(number=w978) -> (single precision float=w976:sgl[])
                n317 = Multiply(x=w987, y=w976) -> (x*y=w988:sgl[])
                n318 = Subtract(x=w986, y=w988) -> (x-y=w983:sgl[])
                n319 = Bundle By Name(cluster=w984, "Signal"=w983) -> (w989:T10)
                n320 = Enqueue Element "Send/Push Data Out"(queue=w985, element=w989) -> ()  [unwired: 2 in, 3 out]
                n321 = disable-structure shown="Enabled" {
                  disable-tunnel: w980 -> [w991 _]
                  disable-tunnel: w979 -> [w990 _]
                  frame Disabled {
                    n322 = Bundle By Name(cluster=w990, "cSegment"=w991) -> ()  [unwired: 1 out]
                  }
                  frame Enabled {
                  }
                }
              }
              frame "Normal" {
                # "dont remember why"
                n323 = Array Subset(array=w1003, length=w992) -> (w993:u8[])  [unwired: 1 in]
                n324 = To Single Precision Float(number=w993) -> (single precision float=w1001:sgl[])
                n325 = Multiply(x=w1000, y=w1001) -> (x*y=w1002:sgl[])
                n326 = Subtract(x=w999, y=w1002) -> (x-y=w996:sgl[])
                n327 = Bundle By Name(cluster=w997, "Signal"=w996) -> (w1004:T10)
                n328 = Enqueue Element "Send/Push Data Out"(queue=w998, element=w1004) -> ()  [unwired: 2 in, 3 out]
                n329 = disable-structure shown="Disabled" {
                  disable-tunnel: w995 -> [w1006 _]
                  disable-tunnel: w994 -> [w1005 _]
                  frame Disabled {
                    n330 = Bundle By Name(cluster=w1005, "cSegment"=w1006) -> ()  [unwired: 1 out]
                  }
                  frame Enabled {
                  }
                }
              }
              frame "MultiRecord" {
                n331 = Multiply(x=0.0 ("y"), y=w1033) -> (x*y=w1015:dbl[])
                n332 = call "EncoderData_Receiver.vi"("Option"=w1018, "Timeout"=50000, "SecondaryDataVIRef"=w1019, "EncoderData queue in"=w1012, "Gage CtrlQueue in"=w1008) -> ("PositionArray"=w1022:dbl[][])  [unwired: 5 in, 1 out]
                n333 = disable-structure shown="Enabled" {
                  disable-tunnel: [w1041 w1042] -> w1029
                  disable-tunnel: w1028 -> [w1040 w1042]
                  frame Enabled {
                    n334 = Enqueue Element ("Send/Push Data Out")(queue=w1040, element=T10 {"tickcount"=0, "Signal"=[], "SecondaryData"=[-inf], "Flag"=enum."LineStart", "Segment#"=1}) -> (queue out=w1041:refnum<queue>)  [unwired: 2 in, 2 out]
                  }
                  frame Disabled {
                  }
                }
                n335 = To Unsigned Long Integer(number=w1015) -> (unsigned 32bit integer=w1017:u32[])
                n336 = flat-sequence {
                  tunnel: [w1044] -> w1009
                  tunnel: w1022 -> [w1043]
                  tunnel: [w1043] -> w1007
                  frame #0 {
                    n337 = call <vilib>:"High Resolution Relative Seconds.vi"() -> ("relative seconds"=w1044:dbl)
                  }
                }
                n338 = for "Voltage converson \nfor compatibility with other hardware" {
                  N: w1021 -> [_]
                  tunnel: w1034 -> [w1060]
                  shift-right: [w1058] -> w1020
                  shift-left: w1023 -> [w1057]
                  tunnel: w1032 -> [w1056]
                  tunnel: w1031 -> [w1055]
                  tunnel: w1030 -> [w1054]
                  shift-right: [w1052] -> w1027
                  shift-left: w1029 -> [w1051]
                  tunnel: w1024 -> [w1049]
                  tunnel: w1007 -> [w1047] mode=indexing
                  tunnel: w1017 -> [w1048] mode=indexing
                  tunnel: [w1047] -> w1010
                  i -> [w1053]
                  n339 = call "VoltDecode-AdvMultiRec.vi"("Adj.SegmentSize"=w1049, "Offset"=w1054, "Slope"=w1055, "Depth"=w1056, "Channels"=1, "cSegment"=w1053, "Buffer In"=w1057) -> ("Data (V)"=w1059:sgl[], "Buffer Out"=w1058:u8[])  [unwired: 3 in]
                  n340 = Bundle By Name(cluster=w1060, "Signal"=w1059, "tickcount"=w1048, "SecondaryData"=w1047, "Segment#"=1) -> (w1061:T10)
                  n341 = Enqueue Element ("Send/Push Data Out")(queue=w1051, element=w1061) -> (queue out=w1052:refnum<queue>)  [unwired: 2 in, 2 out]
                }
                n342 = property class="Arr (strict)"(reference="Encoder feedback ref", "Value"=w1010) -> ()  [unwired: 1 in, 2 out]
                n343 = disable-structure shown="Enabled" {
                  disable-tunnel: w1027 -> [w1036 w1038]
                  disable-tunnel: [w1035 w1038] -> w1013
                  frame Enabled {
                    n344 = Enqueue Element ("Send/Push Data Out")(queue=w1036, element=T10 {"tickcount"=0, "Signal"=[], "SecondaryData"=[inf], "Flag"=enum."LineEnd", "Segment#"=1}) -> (queue out=w1035:refnum<queue>)  [unwired: 2 in, 2 out]
                  }
                  frame Disabled {
                  }
                }
                n345 = flat-sequence {
                  tunnel: [w1045] -> w1026
                  tunnel: w1013 -> [_]
                  frame #0 {
                    n346 = call <vilib>:"High Resolution Relative Seconds.vi"() -> ("relative seconds"=w1045:dbl)
                  }
                }
                n347 = Subtract(x=w1026, y=w1009) -> (x-y=→"volt conv. time":dbl)
                "pos_raw_data" <- w1007
              }
              frame "HwAverage" {
                # "Not implemented"
              }
            }
          }
          frame "GetStat_" {
            n348 = Variant To Data(error in=w1069, type=refnum<queue> refnum ("queue out"), Variant=w1070) -> (data=w1072:refnum<queue>, error out=w1071:errorcluster)
            n349 = Enqueue Element "Send Core Stat"(queue=w1072, element=w1064, error in (no error)=w1071) -> (error out=w1068:errorcluster)  [unwired: 1 in, 2 out]
          }
          frame "GetConfig_" {
            # "solution:\n\n1 call vi ref, vi send out typed command. => possible, idea, time consuming \n\n2 make this frame specific, bad. \n\n3 user event call and wait, then send typed command.  possible, fast?"
            n350 = Variant To Data(type=refnum<queue> refnum ("queue out"), Variant=w1083) -> (data=w1082:refnum<queue>, error out=w1081:errorcluster)  [unwired: 1 in]
            n351 = case shown="No Error" w1081 {
              selector: w1081 -> [_ w1091]
              tunnel: w1082 -> [w1090 _]
              tunnel: w1080 -> [w1087 _]
              tunnel: [w1089 w1091] -> w1079
              tunnel: w1078 -> [w1088 _]
              frame No Error {
                # "short term solution, need refine\nget real result from device"
                n352 = Enqueue Element(queue=w1090, element=w1087, error in (no error)=w1088) -> (error out=w1089:errorcluster)  [unwired: 1 in, 2 out]
              }
              frame Error {
              }
            }
          }
          frame "==ModeSetup==" {
            # "Invalid Frame"
            n353 = xnode "Error Ring"() -> ("error out"=w1094:errorcluster)
          }
          frame "SetSignalBuffer_" {
            n354 = Variant To Data(type=w1111, Variant=w1113) -> (data=w1110:refnum<queue>, error out=w1107:errorcluster)  [unwired: 1 in]
            n355 = Select(t=w1111, s=w1107, f=w1110) -> (s? t:f=w1112:refnum<queue>)
            n356 = xnode "Error Ring"() -> ("error out"=w1106:errorcluster)
            n357 = Select(t=w1106, s=w1107, f=w1108) -> (s? t:f=w1109:errorcluster)
          }
          frame "SetMode_" {
            n358 = Unbundle By Name(w1134) -> ("Mode(Gage)"=w1132:T12, "Handle"=w1125:T13, "SecondaryDataVIRef"=w1124:refnum<vi>, "Option(SecondaryDataVI)"=w1123:i32)
            n359 = Variant To Data(error in=w1129, type=w1132, Variant=w1133) -> (data=w1131:T12, error out=w1130:errorcluster)
            n360 = Select(t=w1132, s=w1130, f=w1131) -> (s? t:f=w1126:T12)
            n361 = Bundle By Name(cluster=w1134, "Mode(Gage)"=w1126) -> (w1135:T4)
            n362 = case shown="\"MultiRecord\", \"HwAverage\"" w1126 {
              tunnel: w1125 -> [w1143 _]
              tunnel: w1122 -> [w1141 _]
              tunnel: w1124 -> [w1140 _]
              tunnel: w1123 -> [w1139 _]
              frame "MultiRecord", "HwAverage" {
                # "for multirecord  and hwaverage"
                n363 = Not A Number/Path/Refnum?(number/path/refnum=w1140) -> (NaN/Path/Refnum?=w1142:bool)
                n364 = call <instrlib>:"CsTool-ConfigureTimeStamp.vi"("Handle Cluster"=w1143) -> ()  [unwired: 2 in, 1 out]
                n365 = case shown="False" w1142 {
                  tunnel: w1141 -> [w1149 _]
                  tunnel: w1140 -> [w1148 _]
                  tunnel: w1139 -> [w1147 _]
                  frame False {
                    # "It also clears buffer"
                    n366 = call-by-ref "?"(reference=w1148, "Option"=w1147) -> ("SecondaryData"=w1146:dbl[])  [unwired: 11 in, 2 out]
                    n367 = Bundle By Name(cluster=T9 {"EncoderReadout States"=enum."SetPosition", "Variant"=variant}, "Variant"=w1146) -> (w1150:T9)
                    n368 = Enqueue Element(queue=w1149, element=w1150) -> (queue out=w1145:refnum<queue>)  [unwired: 2 in, 2 out]
                    n369 = Enqueue Element(queue=w1145, element=T9 {"EncoderReadout States"=enum."Start(Flush)", "Variant"=variant}) -> ()  [unwired: 2 in, 3 out]
                  }
                  frame True {
                  }
                }
              }
              frame Default {
              }
            }
          }
          frame "SetSecondaryDataRef._" {
            n370 = Variant To Data(type=T7 {"SecondaryDataVIRef."=refnum, "Option"=0} ("SecondaryDataParams."), Variant=w1156) -> (data=w1154:T7, error out=w1155:errorcluster)  [unwired: 1 in]
            n371 = case shown="No Error" w1155 {
              tunnel: w1153 -> [w1177 w1185]
              tunnel: [w1176 w1185] -> w1158
              tunnel: w1154 -> [w1172 _]
              tunnel: w1153 -> [w1170 _]
              tunnel: [w1165 w1184] -> w1152
              frame No Error {
                n372 = Unbundle By Name(w1170) -> ("SecondaryDataVIRef"=w1168:refnum<vi>)
                n373 = Unbundle By Name(w1172) -> ("SecondaryDataVIRef."=w1164:refnum<vi>, "Option"=w1171:i32)
                n374 = Not A Number/Path/Refnum?(number/path/refnum=w1168) -> (NaN/Path/Refnum?=w1169:bool)
                n375 = case shown="False" w1169 {
                  tunnel: w1168 -> [w1183 _]
                  tunnel: [w1182 _] -> w1167
                  frame False {
                    n376 = Close Reference(reference=w1183) -> (error out=w1182:errorcluster)  [unwired: 1 in]
                  }
                  frame True {
                  }
                }
                n377 = disable-structure shown="Enabled" {
                  disable-tunnel: w1164 -> [w1178 _]
                  frame Disabled {
                    n378 = Not A Number/Path/Refnum?(number/path/refnum=w1178) -> (NaN/Path/Refnum?=w1179:bool)
                    n379 = case shown="False" w1179 {
                      tunnel: [w1180 _] -> _
                      tunnel: w1178 -> [w1181 _]
                      frame False {
                        n380 = call-by-ref "?"(reference=w1181) -> ("SecondaryData"=w1180:dbl[])  [unwired: 12 in, 2 out]
                        n381 = property on="SetPosition" class="Arr (strict)"("Value"=w1180) -> ()  [unwired: 2 in, 2 out]
                      }
                      frame True {
                      }
                    }
                  }
                  frame Enabled {
                  }
                }
                n382 = property class="VI Interface Type 0"(reference=w1164, error in=w1167) -> (reference out=w1174:refnum<vi>, error out=w1166:errorcluster, "Path"=w1175:path)
                n383 = Open VI Reference(type specifier VI Refnum (for type only)=w1174, vi path=w1175, error in (no error)=w1166) -> (vi reference=w1173:refnum<vi>, error out=w1165:errorcluster)  [unwired: 3 in]
                n384 = Bundle By Name(cluster=w1177, "SecondaryDataVIRef"=w1173, "Option(SecondaryDataVI)"=w1171) -> (w1176:T4)
              }
              frame Error {
                n385 = xnode "Error Ring"() -> ("error out"=w1184:errorcluster)
              }
            }
          }
          frame "SetDynamicBuffer_" {
            (unwired) T23 {"queue out"=refnum, "queue out"=refnum} ("cluster")
            # "Is feedback needed ?"
            n386 = Variant To Data(type=w1191, Variant=w1197) -> (data=w1195:refnum<queue>, error out=w1196:errorcluster)  [unwired: 1 in]
            n387 = case shown="No Error" w1196 {
              tunnel: w1195 -> [w1203 _]
              tunnel: [_ w1205] -> w1194
              tunnel: [w1203 w1204] -> w1192
              tunnel: w1191 -> [w1202 w1204]
              frame No Error {
                "DynamicBuffer_Bak" <- w1202
              }
              frame Error {
                n388 = xnode "Error Ring"() -> ("error out"=w1205:errorcluster)
              }
            }
          }
          frame "===Sync===" {
          }
          frame "LineStart", "SOL_PassThrough" {
            n389 = Enqueue Element(queue=w1218, element=T10 {"tickcount"=0, "Signal"=[], "SecondaryData"=[-inf], "Flag"=enum."LineStart", "Segment#"=1}) -> ()  [unwired: 2 in, 3 out]
          }
          frame "LineEnd", "EOL_PassThrough" {
            n390 = Enqueue Element(queue=w1227, element=T10 {"tickcount"=0, "Signal"=[], "SecondaryData"=[inf], "Flag"=enum."LineEnd", "Segment#"=1}) -> ()  [unwired: 2 in, 3 out]
          }
          frame "FrameStart" {
            n391 = Unbundle By Name(w1238) -> ("Mode(Gage)"=w1235:T12, "SecondaryDataVIRef"=w1237:refnum<vi>, "Option(SecondaryDataVI)"=w1236:i32)
            n392 = case shown="\"MultiRecord\"" w1235 {
              tunnel: w1237 -> [_ w1250]
              tunnel: w1236 -> [_ w1249]
              tunnel: w1234 -> [_ w1248]
              frame Default {
              }
              frame "MultiRecord" {
                n393 = disable-structure shown="Enabled" {
                  disable-tunnel: w1248 -> [w1253 w1254]
                  disable-tunnel: [w1252 w1254] -> w1246
                  frame Disabled {
                    n394 = Enqueue Element(queue=w1253, element=T9 {"EncoderReadout States"=enum."Stop", "Variant"=variant}) -> (queue out=w1252:refnum<queue>)  [unwired: 2 in, 2 out]
                  }
                  frame Enabled {
                  }
                }
                n395 = Not A Number/Path/Refnum?(number/path/refnum=w1250) -> (NaN/Path/Refnum?=w1247:bool)
                n396 = case shown="False" w1247 {
                  tunnel: [w1263 w1264] -> w1245
                  tunnel: w1246 -> [w1260 w1264]
                  tunnel: w1250 -> [w1259 _]
                  tunnel: w1249 -> [w1258 _]
                  frame False {
                    n397 = call-by-ref "?"(reference=w1259, "Option"=w1258) -> ("SecondaryData"=w1257:dbl[])  [unwired: 11 in, 2 out]
                    n398 = Bundle By Name(cluster=T9 {"EncoderReadout States"=enum."SetPosition", "Variant"=variant}, "Variant"=w1257) -> (w1261:T9)
                    n399 = Enqueue Element(queue=w1260, element=w1261) -> (queue out=w1263:refnum<queue>)  [unwired: 2 in, 2 out]
                  }
                  frame True {
                  }
                }
                n400 = disable-structure shown="Enabled" {
                  disable-tunnel: w1245 -> [w1256 _]
                  frame Disabled {
                    n401 = Enqueue Element(queue=w1256, element=T9 {"EncoderReadout States"=enum."Start(Flush)", "Variant"=variant}) -> ()  [unwired: 2 in, 3 out]
                  }
                  frame Enabled {
                  }
                }
              }
            }
          }
          frame Default {
          }
        }
      }
      frame Error {
        n402 = xnode "Error Ring"() -> ("error out"=w1274:errorcluster)
      }
    }
    n403 = call <userlib>:"ErrorLog.vi"("error in (no error)"=w78) -> ("error out"=w71:errorcluster)  [unwired: 10 in]
  }
  "error out" <- w31
  n404 = while {
    tunnel: w38 -> [w1292]
    tunnel: w23 -> [w1291]
    tunnel: w36 -> [w1290]
    tunnel: w28 -> [w1289]
    tunnel: [w1288] -> w26
    tunnel: [w1287] -> _
    tunnel: [w1286] -> _
    stop <- w1286 stop-if-true
    w1285 = 500  # Should not be -1, or do not quit as subVI
    n405 = event shown="[1] \"Gage_Config.Acquisition\": Value Change" {
      selector: _ -> [_ _ _ _ _ _ _ _ _ _ _ _ _ _ _ _]
      dyn-events: _ -> [_ _ _ _ _ _ _ _ _ _ _ _ _ _ _ _]
      timeout: w1285 -> [_ _ _ _ _ _ _ _ _ _ _ _ _ _ _ _]
      tunnel: w1292 -> [w1303 w1320 w1324 w1328 w1333 w1335 w1343 w1347 w1349 w1351 w1353 w1355 w1357 w1359 w1361 w1363]
      tunnel: w1291 -> [_ _ _ _ w1330 _ _ _ _ _ _ _ _ _ _ _]
      tunnel: w1290 -> [w1302 _ _ _ _ _ _ _ _ _ _ _ _ _ _ _]
      tunnel: [_ _ _ _ _ _ TRUE _ _ _ _ _ _ _ _ _] -> w1287
      tunnel: [w1301 _ _ _ _ _ errorcluster {"status"=FALSE, "code"=0, "source"=""} ("error constant") _ _ _ _ _ _ _ _ _] -> w1288
      tunnel: w1285 -> [w1293 _ _ _ _ _ _ _ _ _ _ _ _ _ _ _]
      event Timeout {
        n406 = event-data() -> ()  [unwired: 1 in, 1 out]
        n407 = Bundle By Name(cluster=T3 {"GenericDAQ State"=enum."GetStat_", "Variant"=variant} ("element"), "Variant"=w1302) -> (w1299:T3)
        n408 = Enqueue Element At Opposite End "To get LiveStat,\nIt has to be opposite end"(queue=w1303, element=w1299) -> (error out=w1298:errorcluster)  [unwired: 2 in, 2 out]
        n409 = Dequeue Element(queue=w1302, timeout in ms (-1)=200, error in (no error)=w1298) -> (element=w1297:T4, timed out?=w1295:bool, error out=w1301:errorcluster)  [unwired: 1 out]
        n410 = case shown="True" w1295 {
          tunnel: w1297 -> [w1312 w1316]
          tunnel: [w1311 w1315] -> w1296
          tunnel: w1293 -> [w1307 _]
          frame False {
            n411 = Unbundle By Name(w1312) -> ("TrigCount"=w1310:i32)
            n412 = feedback-in #1(w1310) -> ()
            n413 = feedback #1(0 ("TrigCount")) -> (w1309:i32)
            n414 = Subtract(x=w1310, y=w1309) -> (x-y=w1308:i32)
            n415 = Compound Arithmetic op=MULTIPLY(w1308, invert w1307, 1000.0 ("value")) -> (w1305:dbl)
            n416 = Bundle By Name(cluster=w1312, "TrigRate(Hz)"=w1305) -> (w1311:T4)
          }
          frame True {
            n417 = Bundle By Name(cluster=w1316, "Model"="Gage Busy", "TrigRate(Hz)"=nan) -> (w1315:T4)
          }
        }
        "LiveStat" <- w1296
      }
      event Value Change {
        n418 = event-data() -> ("NewVal"=w1317:T14)  [unwired: 1 in]
        n419 = Bundle By Name(cluster=T3 {"GenericDAQ State"=enum."SetAcquisition_", "Variant"=variant} ("element"), "Variant"=w1317) -> (w1318:T3)
        n420 = Enqueue Element(queue=w1320, element=w1318) -> ()  [unwired: 2 in, 3 out]
      }
      event Value Change {
        n421 = event-data() -> ("NewVal"=w1321:T16)  [unwired: 1 in]
        n422 = Bundle By Name(cluster=T3 {"GenericDAQ State"=enum."SetChannels_", "Variant"=variant} ("element"), "Variant"=w1321) -> (w1322:T3)
        n423 = Enqueue Element(queue=w1324, element=w1322) -> ()  [unwired: 2 in, 3 out]
      }
      event Value Change {
        n424 = event-data() -> ("NewVal"=w1325:T18)  [unwired: 1 in]
        n425 = Bundle By Name(cluster=T3 {"GenericDAQ State"=enum."SetTrigger_", "Variant"=variant} ("element"), "Variant"=w1325) -> (w1326:T3)
        n426 = Enqueue Element(queue=w1328, element=w1326) -> ()  [unwired: 2 in, 3 out]
      }
      event "ConfigAll": Value Change {
        n427 = event-data() -> ()  [unwired: 1 in, 1 out]
        n428 = property class="Clust (strict)"(reference=w1330) -> ("Value"=w1329:T24)  [unwired: 1 in, 2 out]
        n429 = Bundle By Name(cluster=T3 {"GenericDAQ State"=enum."SetAll_AcquChTrig_", "Variant"=variant} ("element"), "Variant"=w1329) -> (w1331:T3)
        n430 = Enqueue Element(queue=w1333, element=w1331) -> ()  [unwired: 2 in, 3 out]
      }
      event "Get_ConfigAll": Value Change {
        n431 = event-data() -> ()  [unwired: 1 in, 1 out]
        n432 = for {
          tunnel: w1335 -> [w1339]
          shift-right: [w1338] -> _
          shift-left: _ -> [w1337]
          tunnel: T3[] [{"GenericDAQ State"=enum."GetAcquisition", "Variant"=variant}, {"GenericDAQ State"=enum."GetChannels", "Variant"=variant}, {"GenericDAQ State"=enum."GetTrigger", "Variant"=variant}] -> [w1336] mode=indexing
          n433 = Enqueue Element(queue=w1339, element=w1336, error in (no error)=w1337) -> (error out=w1338:errorcluster)  [unwired: 1 in, 2 out]
        }
      }
      event "Quit": Value Change {
        n434 = event-data() -> ()  [unwired: 1 in, 1 out]
        n435 = Enqueue Element(queue=w1343, element=T3 {"GenericDAQ State"=enum."Quit", "Variant"=variant}) -> ()  [unwired: 2 in, 3 out]
      }
      event Value Change {
        n436 = event-data() -> ("NewVal"=w1344:T12)  [unwired: 1 in]
        n437 = Bundle By Name(cluster=T3 {"GenericDAQ State"=enum."SetMode_", "Variant"=variant} ("element"), "Variant"=w1344) -> (w1345:T3)
        n438 = Enqueue Element(queue=w1347, element=w1345) -> ()  [unwired: 2 in, 3 out]
      }
      event "fConfig": Value Change {
        n439 = event-data() -> ()  [unwired: 1 in, 1 out]
        n440 = Enqueue Element(queue=w1349, element=T3 {"GenericDAQ State"=enum."fConfigurate", "Variant"=variant}) -> ()  [unwired: 2 in, 3 out]
      }
      event "Start": Value Change {
        n441 = event-data() -> ()  [unwired: 1 in, 1 out]
        n442 = Enqueue Element(queue=w1351, element=T3 {"GenericDAQ State"=enum."fStart", "Variant"=variant}) -> ()  [unwired: 2 in, 3 out]
      }
      event "Reset": Value Change {
        n443 = event-data() -> ()  [unwired: 1 in, 1 out]
        n444 = Enqueue Element(queue=w1353, element=T3 {"GenericDAQ State"=enum."Quit", "Variant"=variant}) -> ()  [unwired: 2 in, 3 out]
      }
      event "CloseAll": Value Change {
        n445 = event-data() -> ()  [unwired: 1 in, 1 out]
        n446 = Enqueue Element(queue=w1355, element=T3 {"GenericDAQ State"=enum."CloseAll", "Variant"=variant}) -> ()  [unwired: 2 in, 3 out]
      }
      event "Close": Value Change {
        n447 = event-data() -> ()  [unwired: 1 in, 1 out]
        n448 = Enqueue Element(queue=w1357, element=T3 {"GenericDAQ State"=enum."Close", "Variant"=variant}) -> ()  [unwired: 2 in, 3 out]
      }
      event "Open": Value Change {
        n449 = event-data() -> ()  [unwired: 1 in, 1 out]
        n450 = Enqueue Element(queue=w1359, element=T3 {"GenericDAQ State"=enum."Open", "Variant"=variant}) -> ()  [unwired: 2 in, 3 out]
      }
      event "Enumerate": Value Change {
        n451 = event-data() -> ()  [unwired: 1 in, 1 out]
        n452 = Enqueue Element(queue=w1361, element=T3 {"GenericDAQ State"=enum."Enumerate", "Variant"=variant}) -> ()  [unwired: 2 in, 3 out]
      }
      event "StartAll": Value Change {
        n453 = event-data() -> ()  [unwired: 1 in, 1 out]
        n454 = property on="Gage_Config" class="Clust (strict)"() -> ("Value"=w1362:T24)  [unwired: 2 in, 2 out]
        n455 = Bundle By Name(cluster=T3 {"GenericDAQ State"=enum."SetAll_AcquChTrig_", "Variant"=variant} ("element"), "Variant"=w1362) -> (w1367:T3)
        n456 = Build Array(T3 {"GenericDAQ State"=enum."Enumerate", "Variant"=variant} ("element"), T3 {"GenericDAQ State"=enum."Open", "Variant"=variant} ("element"), w1367, T3 {"GenericDAQ State"=enum."fConfigurate", "Variant"=variant} ("element"), T3 {"GenericDAQ State"=enum."fStart", "Variant"=variant} ("element")) -> (w1370:T3[])
        n457 = for {
          shift-right: [w1374] -> _
          shift-left: w1363 -> [w1375]
          tunnel: w1370 -> [w1373] mode=indexing
          shift-right: [w1372] -> _
          shift-left: _ -> [w1371]
          n458 = Enqueue Element(queue=w1375, element=w1373, error in (no error)=w1371) -> (queue out=w1374:refnum<queue>, error out=w1372:errorcluster)  [unwired: 1 in, 1 out]
        }
      }
    }
    n459 = Or(x=w1287, y=w1289) -> (x .or. y?=w1286:bool)
  }
  n460 = disable-structure shown="NI_DAQmx_EXIST==TRUE" {
    disable-tunnel: w11 -> [w1377 _]
    disable-tunnel: w12 -> [w1376 _]
    frame condition #0 (active) {
      n461 = disable-structure shown="Enabled" {
        disable-tunnel: w1377 -> [w1379 _]
        disable-tunnel: w1376 -> [w1378 _]
        frame Enabled {
          n462 = call "DualEncodersReadoutCore(NI-DAQmx).vi"("Position Out Queue"=w1378, "ctrl queue in"=w1379) -> ()  [unwired: 9 in, 1 out]
        }
        frame Disabled {
        }
      }
    }
    frame condition #1 {
    }
  }
  n463 = while {
    tunnel: w4 -> [w1385]
    stop <- w1382 stop-if-true
    n464 = Get Queue Status(queue=w1385, return elements? (F)=TRUE) -> (error out=w1382:errorcluster, elements=w1384:T3[])  [unwired: 1 in, 6 out]
    n465 = Reverse 1D Array(array=w1384) -> (reversed array=→"ctrl elements":T3[])
    n466 = Wait (ms)(milliseconds to wait=u32 250) -> ()  [unwired: 1 out]
  }
  n467 = Release Queue(queue=w33, error in (no error)=w31) -> (error out=w37:errorcluster)  [unwired: 1 in, 2 out]
  n468 = Release Queue(queue=w38, error in (no error)=w37) -> (error out=w35:errorcluster)  [unwired: 1 in, 2 out]
  n469 = Merge Errors(w26, w35) -> (w27:errorcluster)
  n470 = Release Queue(queue=w36, error in (no error)=w27) -> (error out=w30:errorcluster)  [unwired: 1 in, 2 out]
  n471 = call <vilib>:"Clear Errors.vi"("error in (no error)"=w30, "specific error code to clear (0: all)"=w29) -> ()  [unwired: 4 in, 2 out]
